vi "Autonomous Independent.vi"() -> ()   [LabVIEW 2014]
doc: "This VI is called when autonomous begins, and will automatically be terminated when autonomous ends. You can carry out timed or sensor driven robot movement independently without needing to return to the caller."
uses:
  <vilib>/Rock Robotics/WPI/Relay/WPI_RelayValue.ctl
  AutonEnum.ctl
  AutonEnumGoAround.ctl
  <vilib>/Rock Robotics/WPI/Joystick/WPI_JoystickGetSetRefNum.vi
  Robot Values.vi
  DriveGlobal.vi
  <vilib>/Rock Robotics/WPI/RobotDrive/WPI_RobotDriveArcadeDrive_Standard(NoSaturation).vi
  Auton1ToteEnum.ctl
panel:
  in  "turn output range 5":cluster{"output high":dbl, "output low":dbl}={"output high"=0.6499999999999999, "output low"=-0.65} {"output low" format="%.2f"; "output high" format="%.2f"}
  in  "PID Turn  gains 5":T1={"proportional gain (Kc)"=0.20000000000000004, "integral time (Ti, min)"=0.0, "derivative time (Td, min)"=0.0} {"derivative time (Td, min)" format="%.3f"; "integral time (Ti, min)" format="%.3f"; "proportional gain (Kc)" format="%.3f"}
  out "Total totes 4":i32
  in  "PID Turn  gains 4":T1={"proportional gain (Kc)"=0.20000000000000004, "integral time (Ti, min)"=0.0, "derivative time (Td, min)"=0.0} {"derivative time (Td, min)" format="%.3f"; "integral time (Ti, min)" format="%.3f"; "proportional gain (Kc)" format="%.3f"}
  in  "turn output range 4":cluster{"output high":dbl, "output low":dbl}={"output high"=0.6500000000000001, "output low"=-0.65} {"output low" format="%.2f"; "output high" format="%.2f"}
  out "Total totes 3":i32
  in  "PID Turn  gains 3":T1={"proportional gain (Kc)"=0.05, "integral time (Ti, min)"=0.01, "derivative time (Td, min)"=0.0} {"derivative time (Td, min)" format="%.3f"; "integral time (Ti, min)" format="%.3f"; "proportional gain (Kc)" format="%.3f"}
  in  "turn output range 3":cluster{"output high":dbl, "output low":dbl}={"output high"=0.4, "output low"=-0.4} {"output low" format="%.2f"; "output high" format="%.2f"}
  out "Total totes 2":i32
  in  "PID Turn  gains 2":T1={"proportional gain (Kc)"=0.05, "integral time (Ti, min)"=0.01, "derivative time (Td, min)"=0.0} {"derivative time (Td, min)" format="%.3f"; "integral time (Ti, min)" format="%.3f"; "proportional gain (Kc)" format="%.3f"}
  in  "turn output range 2":cluster{"output high":dbl, "output low":dbl}={"output high"=0.4, "output low"=-0.4} {"output low" format="%.2f"; "output high" format="%.2f"}
  in  "Average gains 2":T1={"proportional gain (Kc)"=0.05, "integral time (Ti, min)"=0.0, "derivative time (Td, min)"=0.0}
  in  "output range":cluster{"output high":dbl, "output low":dbl}={"output high"=0.6, "output low"=-0.6}
  out "Total totes":i32
  out "Totes grabed":i32
  in  "PID Turn  gains":T1={"proportional gain (Kc)"=0.09999999999999999, "integral time (Ti, min)"=0.01, "derivative time (Td, min)"=0.0} {"derivative time (Td, min)" format="%.3f"; "integral time (Ti, min)" format="%.3f"; "proportional gain (Kc)" format="%.3f"}
  in  "turn output range":cluster{"output high":dbl, "output low":dbl}={"output high"=0.7, "output low"=-0.7} {"output low" format="%.2f"; "output high" format="%.2f"}
  in  "Average gains":T1={"proportional gain (Kc)"=0.01, "integral time (Ti, min)"=0.0, "derivative time (Td, min)"=0.0} {"derivative time (Td, min)" format="%.3f"; "integral time (Ti, min)" format="%.4f"; "proportional gain (Kc)" format="%.3f"}
  in  "name or relative path":string
  in  "P2":dbl[][](array[numeric])
  in  "P1":dbl[][](array[numeric])
  out "Current Movement, for debugging":T2 {"Y Joystick Value" scale=1.0..-1.0; "X Joystick Value" scale=-1.0..1.0}
  in  "Array of robot movements":T3(array[cluster]) {"Y Joystick Value" scale=1.0..-1.0; "X Joystick Value" scale=-1.0..1.0}
  # "Be sure to right-click and choose Data Operations>>Make Current Value default if you want to save the array values with the VI"
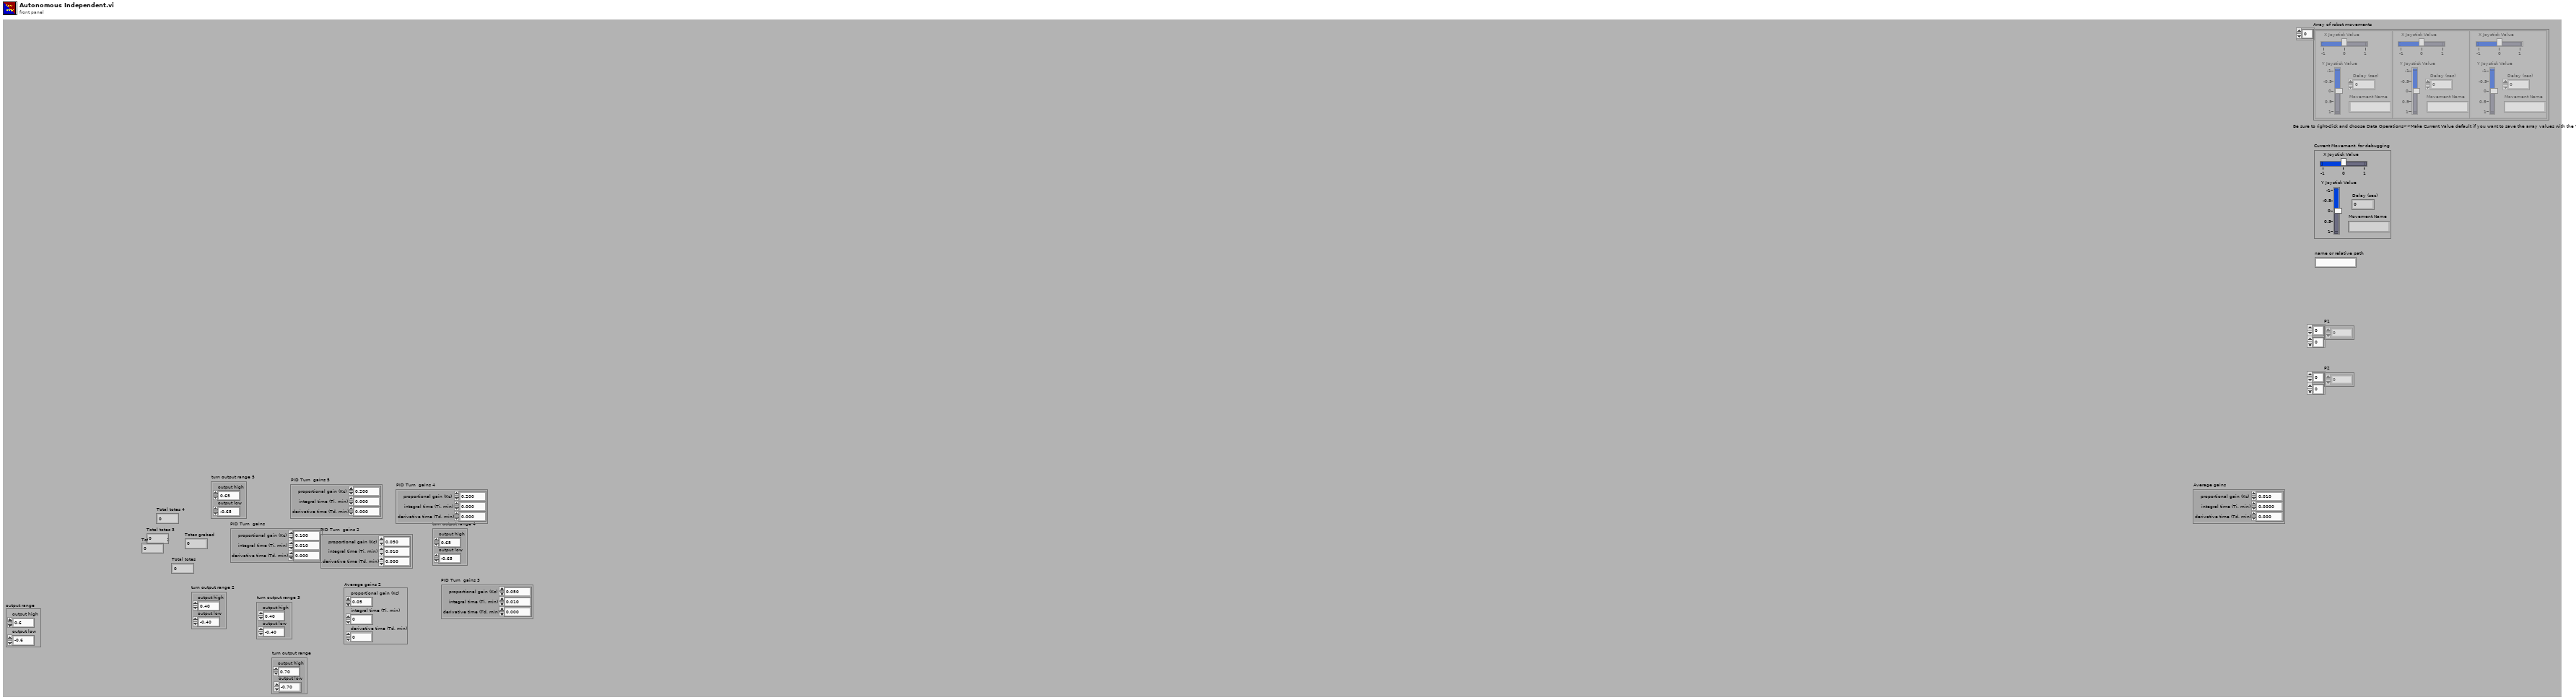
[diagram p1: front panel]
types:
  T1 = cluster{"proportional gain (Kc)":dbl, "integral time (Ti, min)":dbl, "derivative time (Td, min)":dbl}
  T2 = cluster{"X Joystick Value":dbl, "Y Joystick Value":dbl, "Delay (sec)":dbl, "Movement Name":string}
  T3 = cluster{"X Joystick Value":dbl, "Y Joystick Value":dbl, "Delay (sec)":dbl, "Movement Name":string}[]
  T4 = enum16{"Nothing", "Start", "Push", "Finish", "Turn", "Stack"}
  T5 = typedef "WPI_RelayValue.ctl" = enum16{"Off", "On", "Forward", "Reverse"}
  T6 = typedef "AutonEnum.ctl" = enum16{"Go Around", "Nothing", "Start", "Push", "Release Totes", "Turn", "To Auto", "Stack", "Finish"}
  T7 = typedef "AutonEnumGoAround.ctl" = enum16{"Turn Right 1", "Go Straight 1", "Turn Left 1", "Go Straight 2", "Turn Left 2", "Go Straight 3", "Turn Right 3", "Go Straight 4", "Nothing"}
  T8 = typedef "Auton1ToteEnum.ctl" = enum16{"Start", "First Forward", "Get First Tote", "First Pick Up", "Stop"}
  T9 = cluster{"RightMotorSpeed":dbl, "LeftMotorSpeed":dbl}
  T10 = cluster{"Tracking Tote?":bool, "ToteRightSpeed":dbl, "ToteLeftSpeed":dbl, "Drive Encoder reset":bool, "Right Wheel \n(Cm)":dbl, "Left Wheel \n(Cm)":dbl}
  T11 = cluster{"Lift Position":i32, "Lift Speed Override":dbl, "OverrideTele?":bool, "OverrideDash":bool}
  T12 = cluster{"Lift Encoder Height Right (cm)":dbl, "Lift Encoder Height Left (cm)":dbl, "Right Prox":bool, "Left Prox":bool, "Gyro Angle":dbl, "Gyro anglar rate":dbl, "Gyro Reset":bool, "Drive encoder Dash reset":bool}
  T13 = typedef "WPI_JoystickDevRef.ctl" = cluster{"Device":T14}
  T14 = typedef "WPI_JoystickDeviceEnum.ctl" = enum16{"USB 0", "USB 1", "USB 2", "USB 3", "USB 4", "USB 5"}
  T15 = typedef "WPI_RobotDriveDevRef.ctl" = cluster{"DevStatus":errorcluster, "Motors[]":T16[], "Square Inputs":bool, "Max Output":dbl}
  T16 = typedef "WPI_MotorControlDeviceRef.ctl" = cluster{"DeviceStatus":errorcluster, "Type":T17, "PWM":cluster{"Controller":T18, "PWM Channel":T19, "DeadBand":T20}, "CAN":cluster{"Device Number":u8, "Control Mode":T21, "Semaphore":T22, "Max Vout":dbl, "TalonSRX Control Mode":T23}, "Invert":bool, "TransformRef":T24, "InvTransformRef":T24}
  T17 = typedef "WPI_MotorControlType.ctl" = enum16{"PWM", "CAN", "CANTalonSRX"}
  T18 = typedef "FPGA_TypedefDigitalModule.ctl" = enum16{"Controller 1"}
  T19 = typedef "FPGA_DIOPWMChannel.ctl" = enum8{"PWM 0", "PWM 1", "PWM 2", "PWM 3", "PWM 4", "PWM 5", "PWM 6", "PWM 7", "PWM 8", "PWM 9", "PWM MXP 0", "PWM MXP 1", "PWM MXP 2", "PWM MXP 3", "PWM MXP 4", "PWM MXP 5", "PWM MXP 6", "PWM MXP 7", "PWM MXP 8", "PWM MXP 9", "Invalid"}
  T20 = typedef "WPI_PWMDeadband.ctl" = cluster{"Name":string, "maxPositivePwm":i32, "minPositivePwm":i32, "centerPwm":i32, "maxNegativePwm":i32, "minNegativePwm":i32, "angularRange":u16}
  T21 = typedef "WPI_CANJaguar_ControlMode.ctl" = enum8{"Percent VBus", "Current", "Speed", "Position", "Voltage"}
  T22 = typedef "Semaphore RefNum" = refnum<k1>
  T23 = typedef "WPI_CANTalonSRX_APIControlMode.ctl" = enum8{"Percent VBus", "Speed", "Position", "Slave", "Unchanged / Invalid"}
  T24 = typedef "WPI_PWMTransform_ConPane.ctl" = refnum<vi>
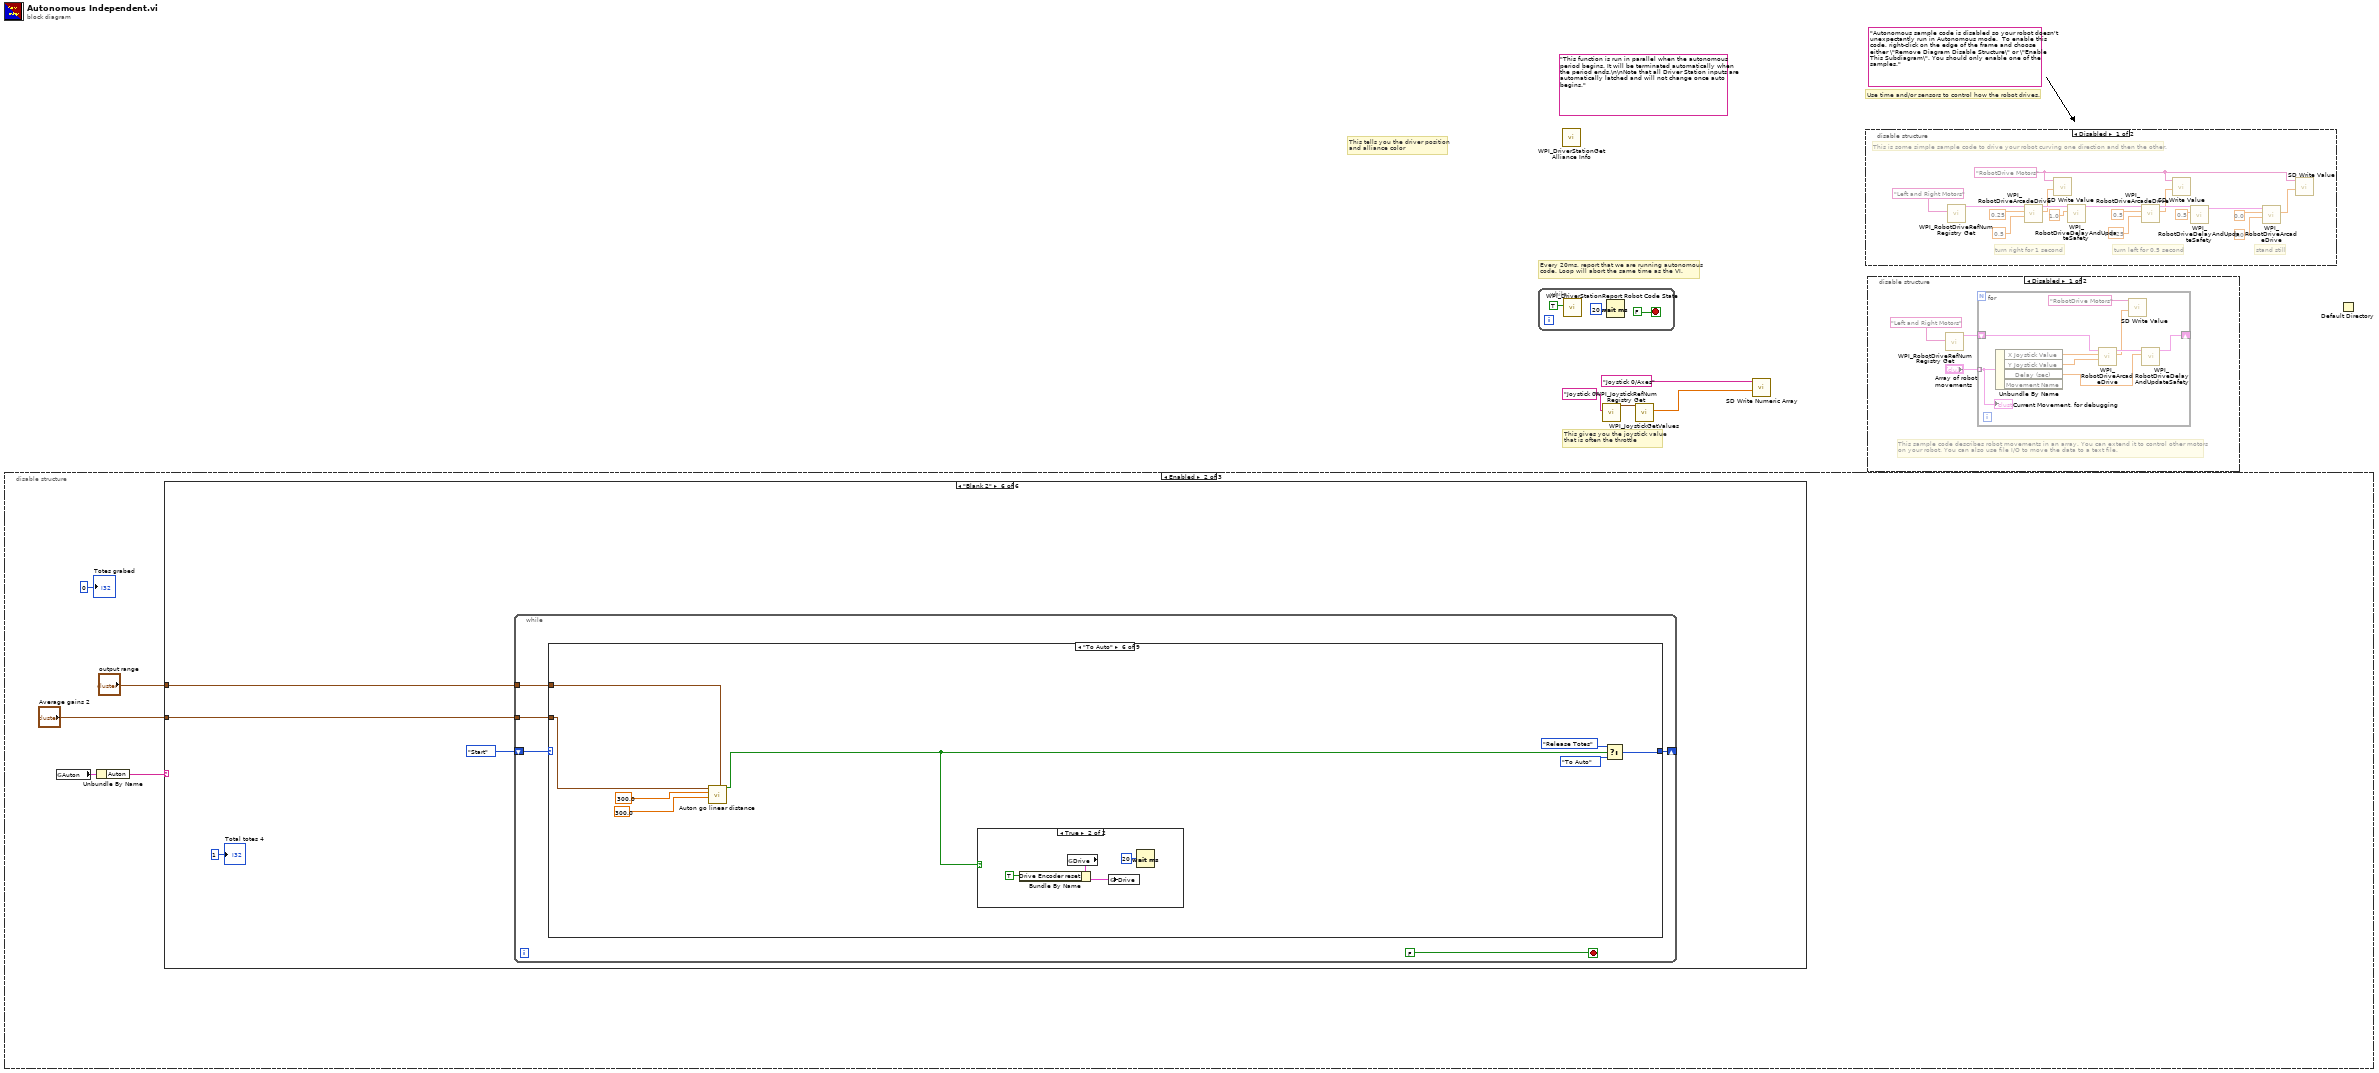
[diagram p0: block diagram]
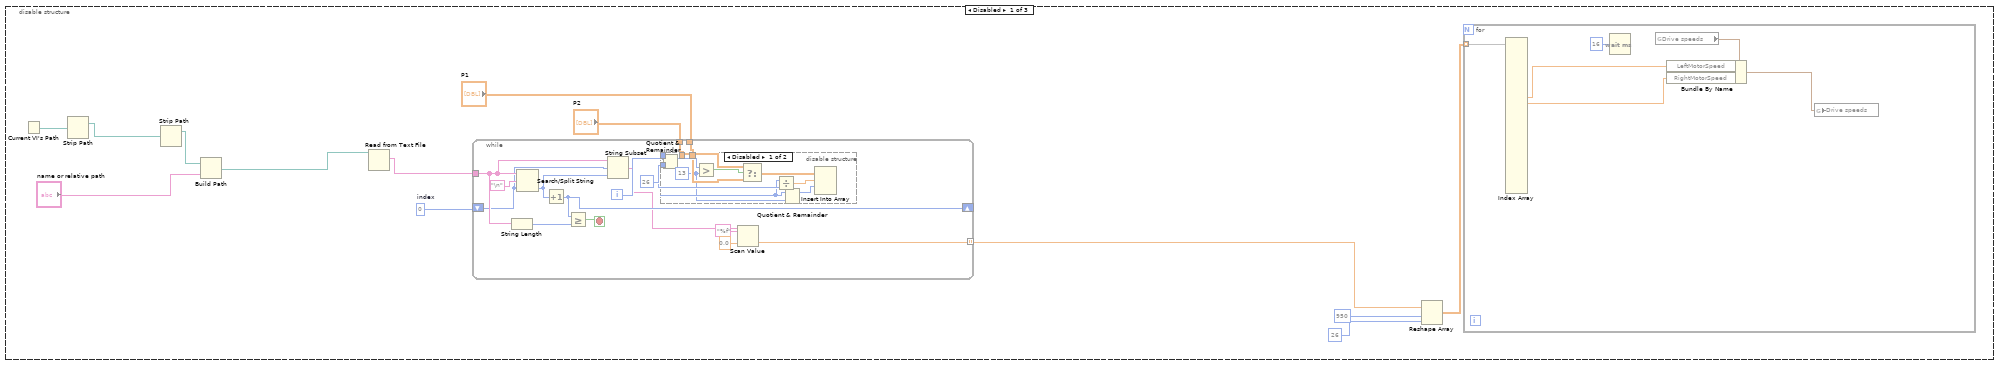
[diagram p2: hidden frame]
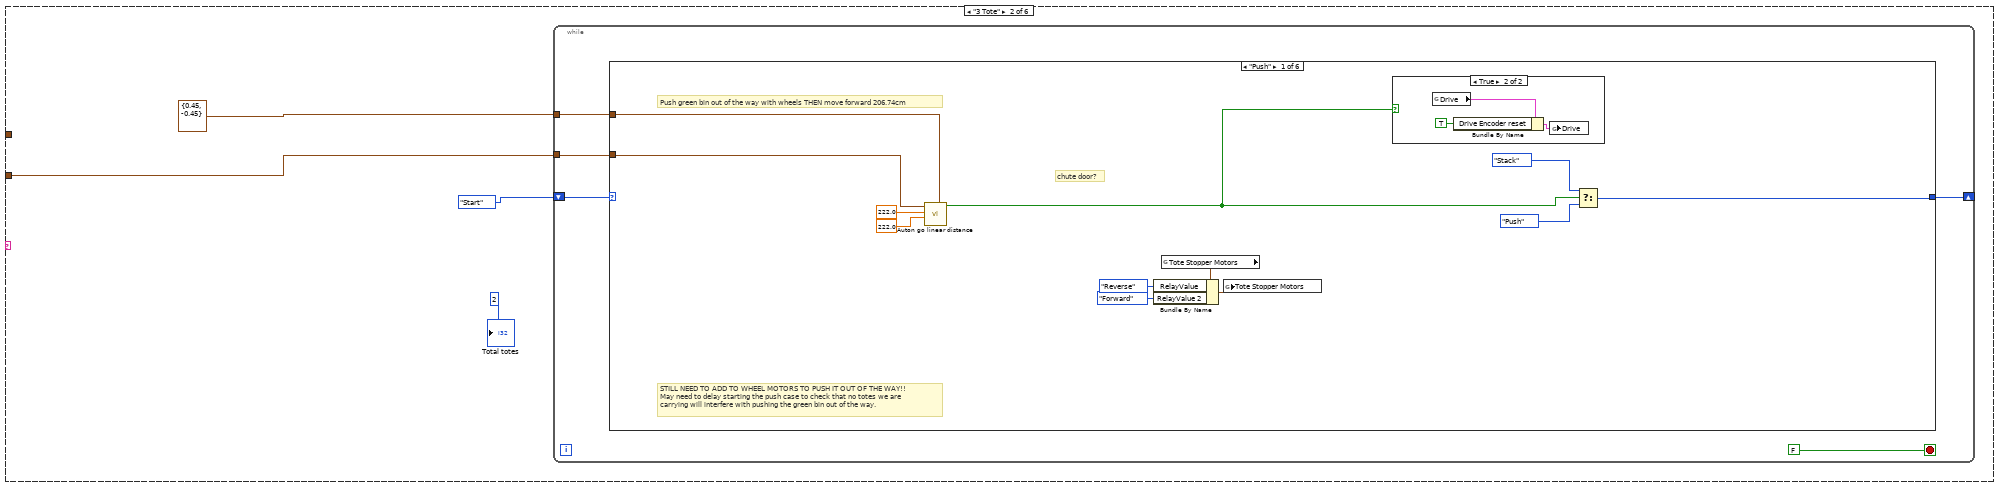
[diagram p5: hidden frame]
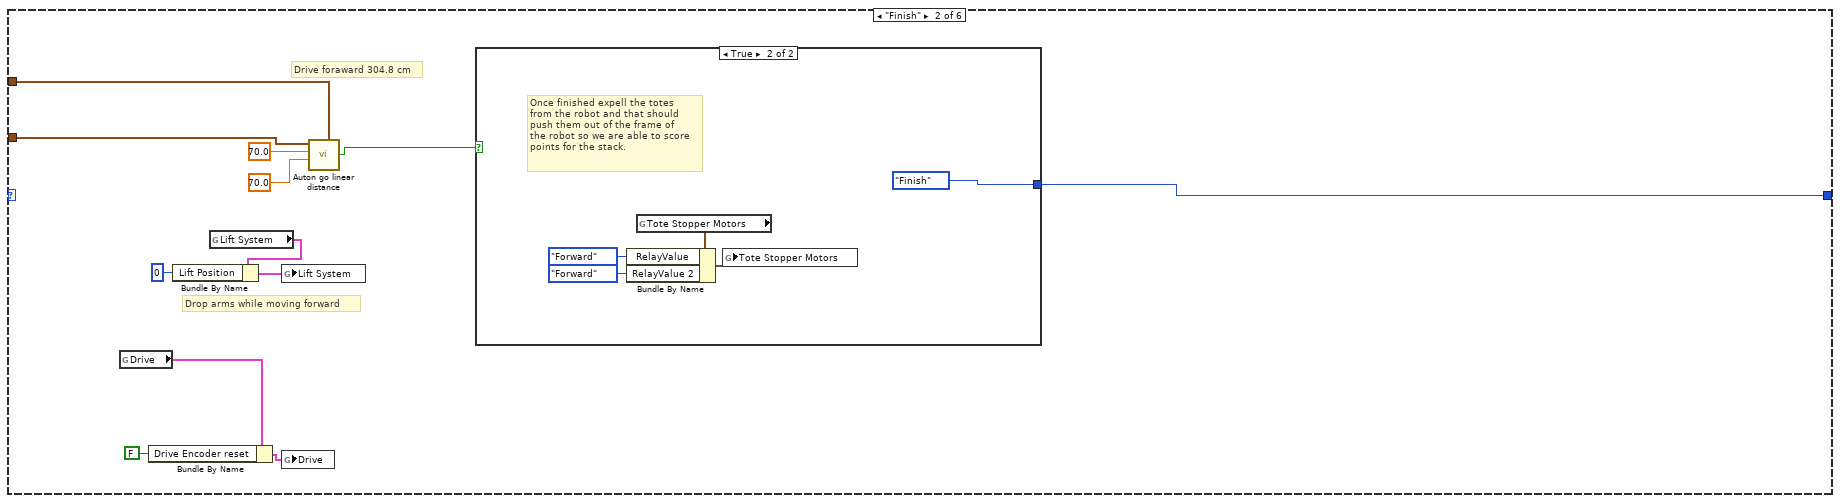
[diagram p7: hidden frame]
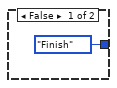
[diagram p8: hidden frame]
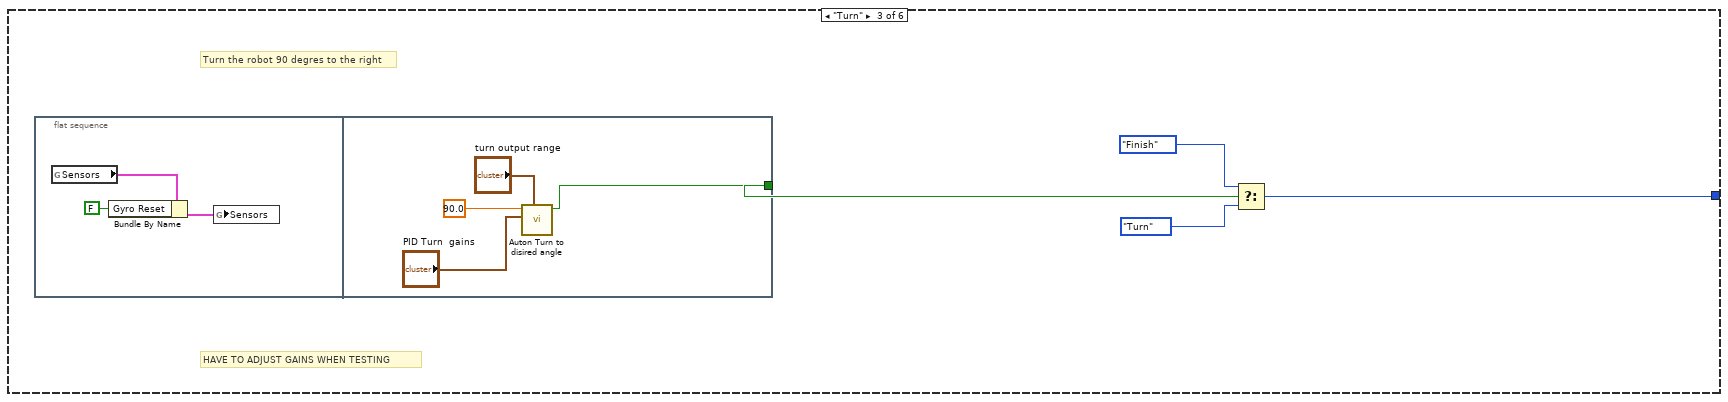
[diagram p9: hidden frame]
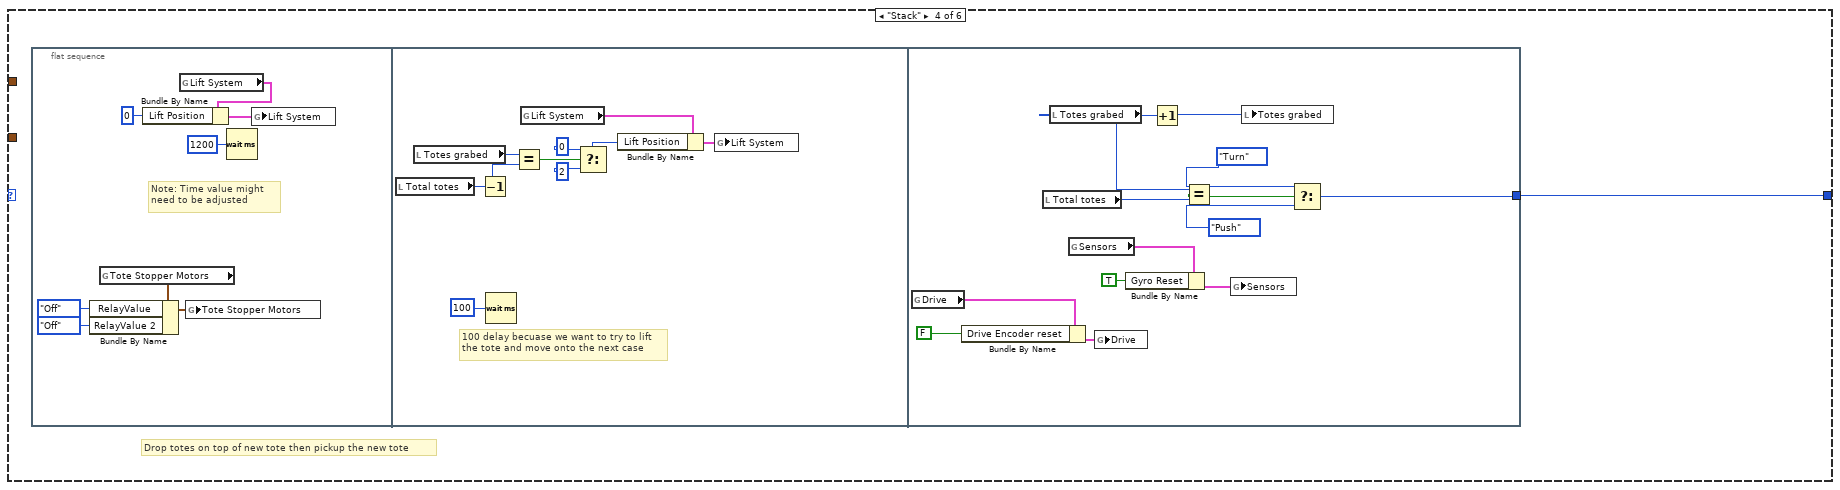
[diagram p10: hidden frame]
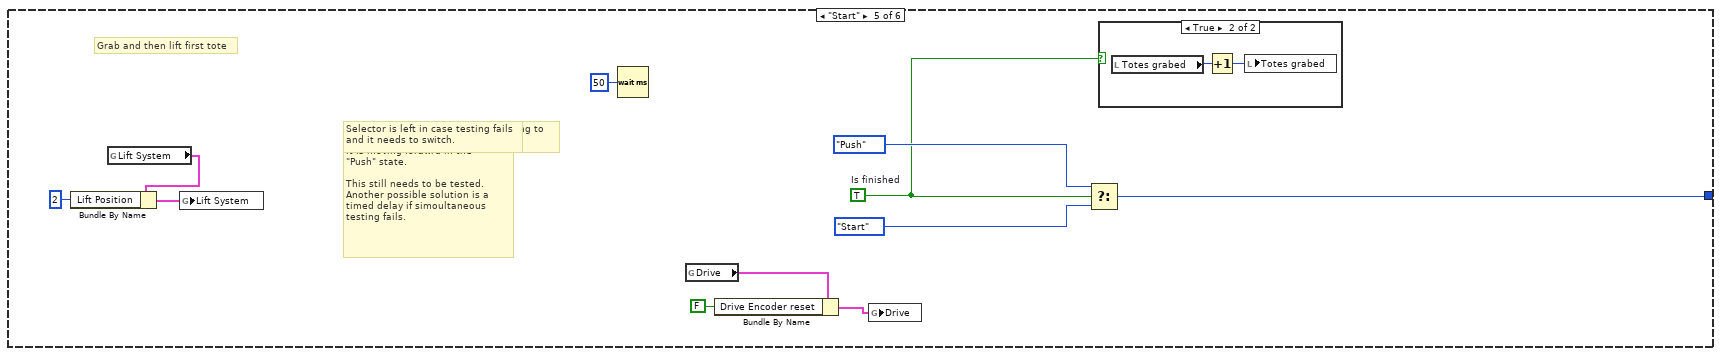
[diagram p11: hidden frame]
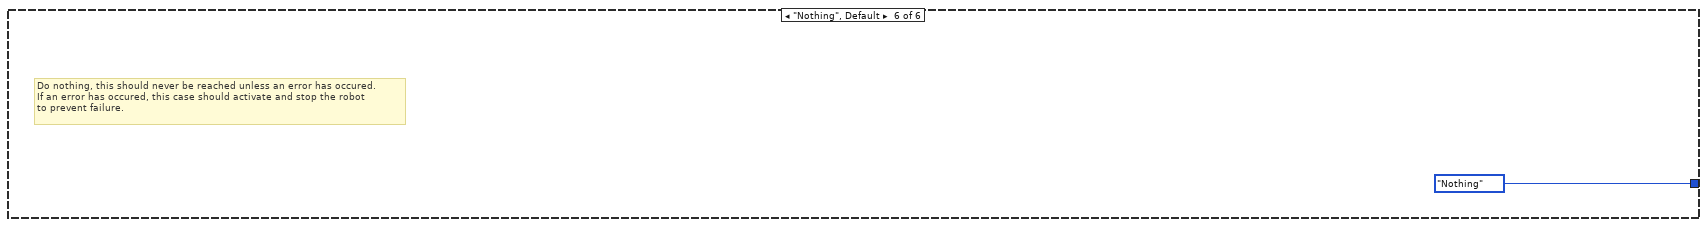
[diagram p13: hidden frame]
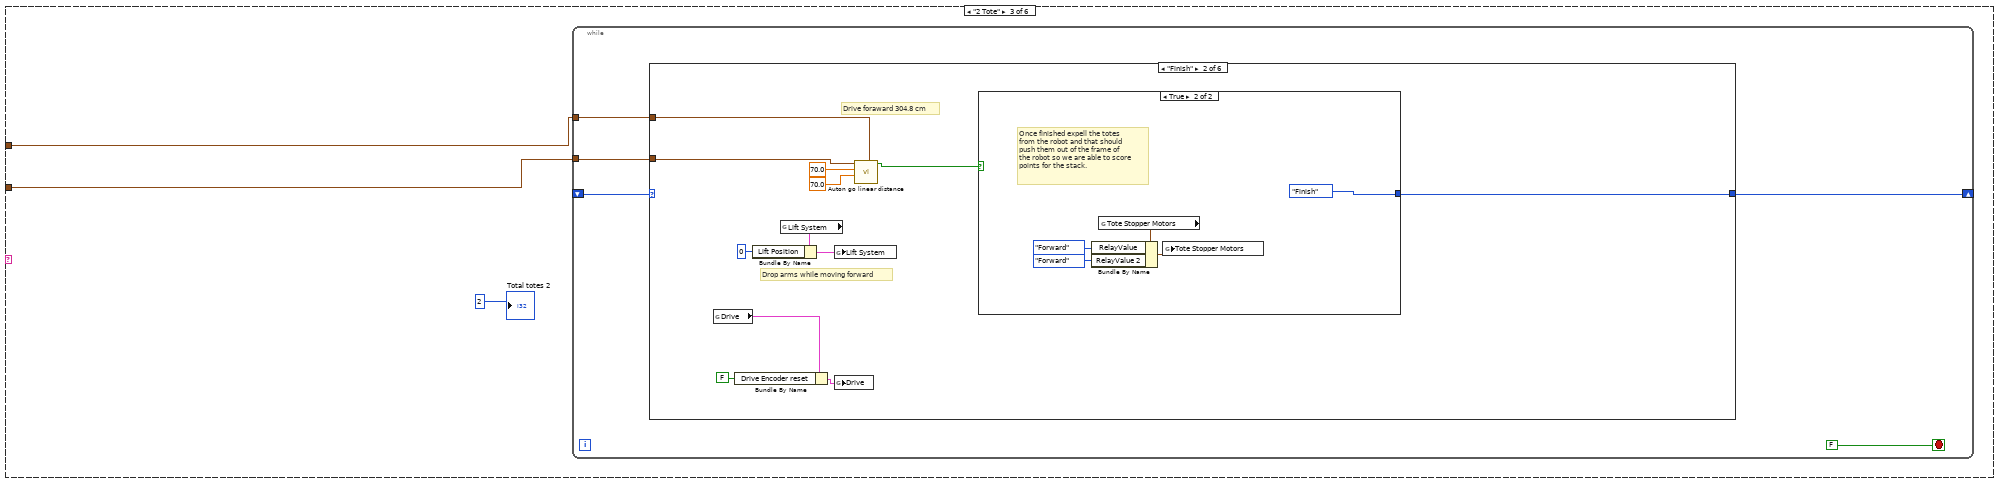
[diagram p14: hidden frame]
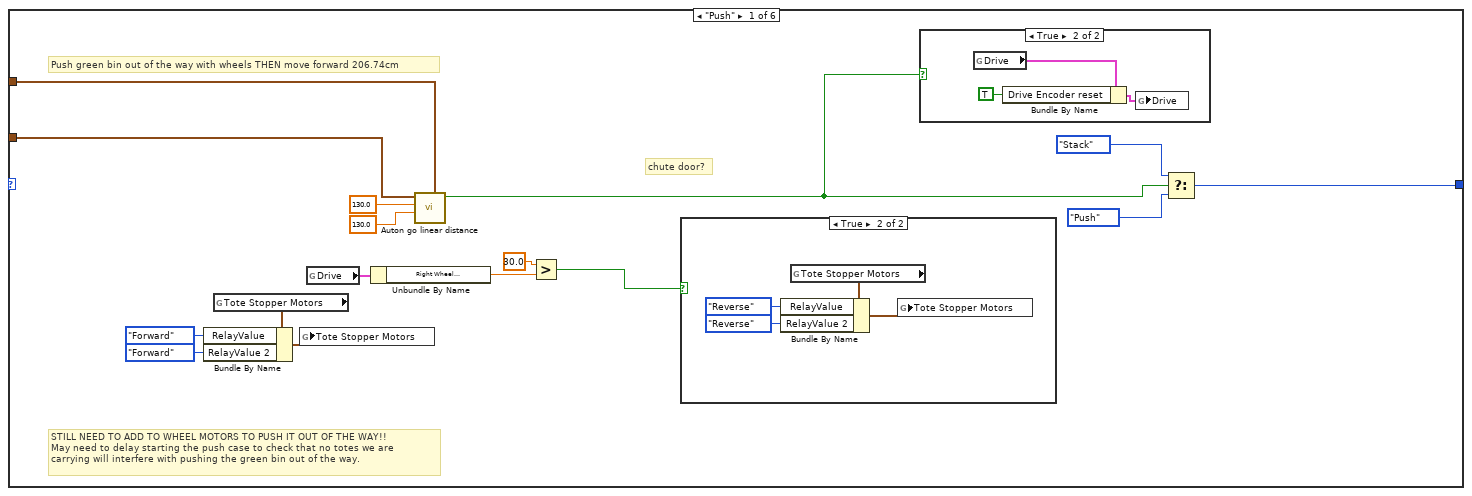
[diagram p15: hidden frame]
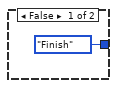
[diagram p18: hidden frame]
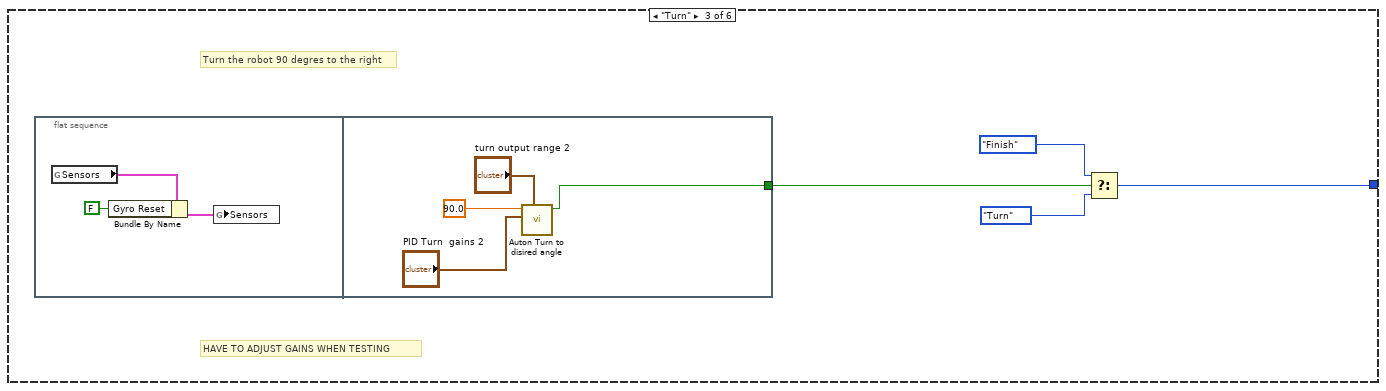
[diagram p19: hidden frame]
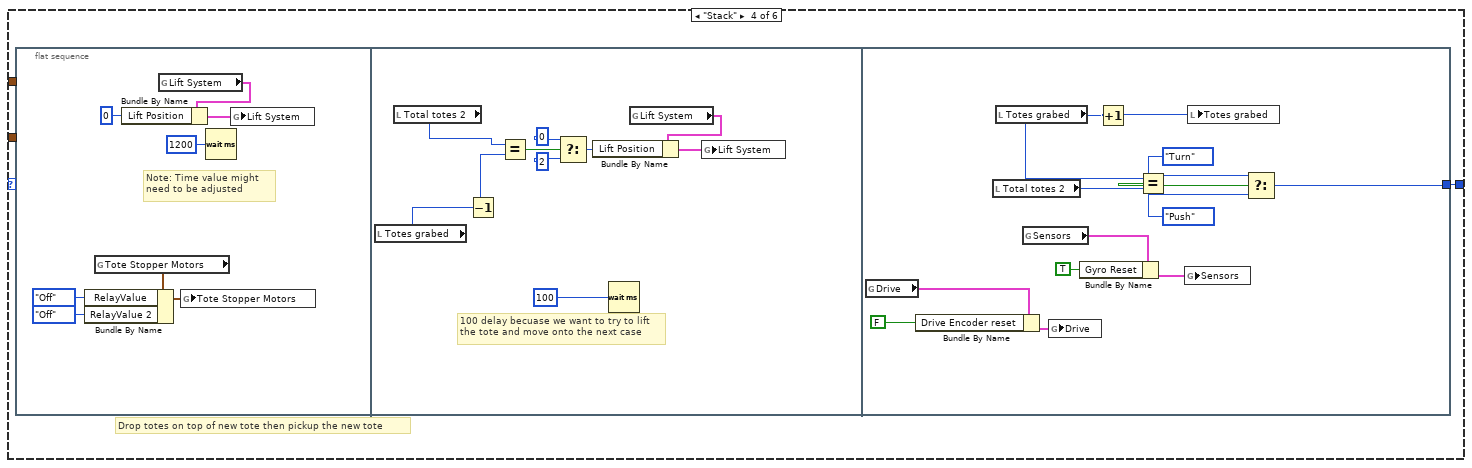
[diagram p20: hidden frame]
diagram:
  (unwired) "Autonomous sample code is disabled so your robot doesn't unexpectantly run in Autonomous mode.  To enable this code, right-click on the edge of the frame and choose either \"Remove Diagram Disable Structure\" or \"Enable This Subdiagram\". You should only enable one of the samples."
  (unwired) "This function is run in parallel when the autonomous period begins. It will be terminated automatically when the period ends.\n\nNote that all Driver Station inputs are automatically latched and will not change once auto begins."
  # "Every 20ms, report that we are running autonomous\ncode. Loop will abort the same time as the VI."
  # "This gives you the joystick value\nthat is often the throttle"
  # "Use time and/or sensors to control how the robot drives."
  # "This tells you the driver position\nand alliance color"
  n1 = disable-structure shown="Enabled" {
    frame Disabled {
      w16 = 0  # index
      n2 = Current VI's Path() -> (path=w10:path)
      n3 = Strip Path(path=w10) -> (stripped path=w9:path)  [unwired: 1 out]
      n4 = Strip Path(path=w9) -> (stripped path=w8:path)  [unwired: 1 out]
      n5 = Build Path(base path=w8, name or relative path="name or relative path") -> (appended path=w7:path)
      n6 = Read from Text File(file (use dialog)=w7) -> (text=w17:string)  [unwired: 3 in, 3 out]
      n7 = while {
        tunnel: w17 -> [w34]
        shift-right: [w35] -> _
        shift-left: w16 -> [w33]
        tunnel: "P1" -> [w30]
        tunnel: "P2" -> [w31]
        tunnel: [w27] -> w13 mode=indexing
        i -> [w28]
        stop <- w37 stop-if-true
        n8 = String Length(string=w34) -> (length=w38:i32)
        n9 = Search/Split String(string=w34, search string/char (-)="\n", offset (0)=w33) -> (offset of match=w32:i32)  [unwired: 2 out]
        n10 = Increment(x=w32) -> (x+1=w35:i32)
        n11 = Greater Or Equal?(x=w35, y=w38) -> (x >= y?=w37:bool)
        n12 = String Subset(string=w34, offset (0)=w33, length (rest)=w32) -> (substring=w26:string)
        n13 = disable-structure shown="Disabled" {
          disable-tunnel: w31 -> [w46 _]
          disable-tunnel: w30 -> [w45 _]
          disable-tunnel: 26 ("y") -> [w42 _]
          disable-tunnel: w28 -> [w40 _]
          frame Disabled {
            w39 = 13 ("y")
            n14 = Quotient & Remainder(x=w40, y=w42) -> (x-y*floor(x/y)=w48:i32)  [unwired: 1 out]
            n15 = Greater?(x=w48, y=w39) -> (0:w47:bool)
            n16 = Select(t=w46, s=w47, f=w45) -> (s? t:f=w44:dbl[][])
            n17 = Divide(x=w40, y=w42) -> (x/y=w43:dbl)
            n18 = Quotient & Remainder(x=w40, y=w39) -> (x-y*floor(x/y)=w41:i32)  [unwired: 1 out]
            n19 = Insert Into Array(array=w44, index (row)=w43, index (col)=w41) -> ()  [unwired: 1 in, 1 out]
          }
          frame Enabled {
          }
        }
        n20 = Scan Value(string=w26, format string="%f", default (0 dbl)=0.0 ("default (0 I32)")) -> (value=w27:dbl)  [unwired: 1 out]
      }
      n21 = Reshape Array(w13, 950 ("dimension size"), 26 ("dimension size")) -> (w5:dbl[][])
      n22 = for {
        tunnel: w5 -> [w23] mode=indexing
        n23 = Index Array(array=w23) -> (element #9=w21:dbl, element #10=w20:dbl)  [unwired: 26 in, 24 out]
        n24 = Wait (ms)(milliseconds to wait=u32 16) -> ()  [unwired: 1 out]
        n25 = global read "DriveGlobal.vi" "Drive speeds"() -> (w19:T9)
        n26 = Bundle By Name(cluster=w19, "LeftMotorSpeed"=w21, "RightMotorSpeed"=w20) -> (w18:T9)
        n27 = global write "DriveGlobal.vi" "Drive speeds"(w18) -> ()
      }
    }
    frame Enabled {
      n28 = global read "Robot Values.vi" "Auton"() -> (w50:cluster{"Auton":string})
      n29 = Unbundle By Name(w50) -> ("Auton"=w49:string)
      n30 = case shown="\"Blank 2\"" w49 {
        tunnel: "Average gains 2" -> [_ w54 w153 w260 w372 w379]
        tunnel: "output range" -> [_ _ w154 w259 w371 w380]
        frame "False", Default {
        }
        frame "3 Tote" {
          n31 = while {
            shift-right: [w61] -> _
            shift-left: T4."Start" -> [w62]
            tunnel: w54 -> [w59]
            tunnel: cluster{"output high":dbl, "output low":dbl} {"output high"=0.45, "output low"=-0.45} ("output range") -> [w58]
            stop <- FALSE stop-if-true
            n32 = case shown="\"Push\"" w62 {
              tunnel: [w72 w81 w97 w107 w147 T4."Nothing"] -> w61
              tunnel: w59 -> [w70 w86 _ _ _ _]
              tunnel: w58 -> [w71 w87 _ _ _ _]
              frame "Push" {
                # "chute door?"
                # "STILL NEED TO ADD TO WHEEL MOTORS TO PUSH IT OUT OF THE WAY!!\nMay need to delay starting the push case to check that no totes we are \ncarrying will interfere with pushing the green bin out of the way."
                # "Push green bin out of the way with wheels THEN move forward 206.74cm"
                n33 = call "Auton go linear distance.vi"("Average gains"=w70, "PID setpoint"=222.0, "Goal"=222.0, "output range"=w71) -> ("Done?"=w68:bool)  [unwired: 4 in]
                n34 = global read "Robot Values.vi" "Tote Stopper Motors"() -> (w64:cluster{"RelayValue":T5, "RelayValue 2":T5})
                n35 = Bundle By Name(cluster=w64, "RelayValue"=WPI_RelayValue."Reverse", "RelayValue 2"=WPI_RelayValue."Forward") -> (w63:cluster{"RelayValue":T5, "RelayValue 2":T5})
                n36 = global write "Robot Values.vi" "Tote Stopper Motors"(w63) -> ()
                n37 = case shown="True" w68 {
                  frame False {
                  }
                  frame True {
                    n38 = global read "Robot Values.vi" "Drive"() -> (w76:T10)
                    n39 = Bundle By Name(cluster=w76, "Drive Encoder reset"=TRUE) -> (w77:T10)
                    n40 = global write "Robot Values.vi" "Drive"(w77) -> ()
                  }
                }
                n41 = Select(t=T4."Stack", s=w68, f=T4."Push") -> (s? t:f=w72:T4)
              }
              frame "Finish" {
                # "Drop arms while moving forward"
                # "Drive foraward 304.8 cm"
                n42 = global read "Robot Values.vi" "Drive"() -> (w83:T10)
                n43 = Bundle By Name(cluster=w83, "Drive Encoder reset"=FALSE) -> (w84:T10)
                n44 = global read "Robot Values.vi" "Lift System"() -> (w79:T11)
                n45 = Bundle By Name(cluster=w79, "Lift Position"=0) -> (w80:T11)
                n46 = global write "Robot Values.vi" "Lift System"(w80) -> ()
                n47 = global write "Robot Values.vi" "Drive"(w84) -> ()
                n48 = call "Auton go linear distance.vi"("Average gains"=w86, "PID setpoint"=70.0, "Goal"=70.0, "output range"=w87) -> ("Done?"=w85:bool)  [unwired: 4 in]
                n49 = case shown="True" w85 {
                  tunnel: [T4."Finish" T4."Finish"] -> w81
                  frame False {
                  }
                  frame True {
                    # "Once finished expell the totes\nfrom the robot and that should\npush them out of the frame of\nthe robot so we are able to score\npoints for the stack."
                    n50 = global read "Robot Values.vi" "Tote Stopper Motors"() -> (w93:cluster{"RelayValue":T5, "RelayValue 2":T5})
                    n51 = Bundle By Name(cluster=w93, "RelayValue"=WPI_RelayValue."Forward", "RelayValue 2"=WPI_RelayValue."Forward") -> (w94:cluster{"RelayValue":T5, "RelayValue 2":T5})
                    n52 = global write "Robot Values.vi" "Tote Stopper Motors"(w94) -> ()
                  }
                }
              }
              frame "Turn" {
                # "HAVE TO ADJUST GAINS WHEN TESTING"
                # "Turn the robot 90 degres to the right"
                n53 = flat-sequence {
                  tunnel: [w103] -> w96
                  frame #0 {
                    n54 = global read "Robot Values.vi" "Sensors"() -> (w101:T12)
                    n55 = Bundle By Name(cluster=w101, "Gyro Reset"=FALSE) -> (w100:T12)
                    n56 = global write "Robot Values.vi" "Sensors"(w100) -> ()
                  }
                  frame #1 {
                    n57 = call "Auton Turn to disired angle.vi"("Power output range"="turn output range", "PID Turn  gains"="PID Turn  gains", "Angle setpoint"=90.0) -> ("In Range?"=w103:bool)  [unwired: 8 in]
                  }
                }
                n58 = Select(t=T4."Finish", s=w96, f=T4."Turn") -> (s? t:f=w97:T4)
              }
              frame "Stack" {
                # "Drop totes on top of new tote then pickup the new tote"
                n59 = flat-sequence {
                  tunnel: [w138] -> w107
                  frame #0 {
                    # "Note: Time value might \nneed to be adjusted"
                    n60 = global read "Robot Values.vi" "Tote Stopper Motors"() -> (w110:cluster{"RelayValue":T5, "RelayValue 2":T5})
                    n61 = Bundle By Name(cluster=w110, "RelayValue"=WPI_RelayValue."Off", "RelayValue 2"=WPI_RelayValue."Off") -> (w111:cluster{"RelayValue":T5, "RelayValue 2":T5})
                    n62 = global read "Robot Values.vi" "Lift System"() -> (w114:T11)
                    n63 = Bundle By Name(cluster=w114, "Lift Position"=0) -> (w113:T11)
                    n64 = global write "Robot Values.vi" "Tote Stopper Motors"(w111) -> ()
                    n65 = Wait (ms)(milliseconds to wait=u32 1200) -> ()  [unwired: 1 out]
                    n66 = global write "Robot Values.vi" "Lift System"(w113) -> ()
                  }
                  frame #1 {
                    # "100 delay becuase we want to try to lift\nthe tote and move onto the next case"
                    n67 = local read "Total totes"() -> (w118:i32)
                    n68 = local read "Totes grabed"() -> (w116:i32)
                    n69 = Decrement(x=w118) -> (x-1=w117:i32)
                    n70 = Wait (ms)(milliseconds to wait=u32 100) -> ()  [unwired: 1 out]
                    n71 = Equal?(x=w116, y=w117) -> (x = y?=w122:bool)
                    n72 = global read "Robot Values.vi" "Lift System"() -> (w124:T11)
                    n73 = Select(t=0 ("Lift Position"), s=w122, f=2 ("Lift Position")) -> (s? t:f=w119:i32)
                    n74 = Bundle By Name(cluster=w124, "Lift Position"=w119) -> (w125:T11)
                    n75 = global write "Robot Values.vi" "Lift System"(w125) -> ()
                  }
                  frame #2 {
                    n76 = global read "Robot Values.vi" "Drive"() -> (w127:T10)
                    n77 = Bundle By Name(cluster=w127, "Drive Encoder reset"=FALSE) -> (w128:T10)
                    n78 = local read "Total totes"() -> (w135:i32)
                    n79 = local read "Totes grabed"() -> (w137:i32)
                    n80 = global read "Robot Values.vi" "Sensors"() -> (w130:T12)
                    n81 = global write "Robot Values.vi" "Drive"(w128) -> ()
                    n82 = Bundle By Name(cluster=w130, "Gyro Reset"=TRUE) -> (w131:T12)
                    n83 = Increment(x=w137) -> (x+1=w136:i32)
                    n84 = Equal?(x=w136, y=w135) -> (x = y?=w133:bool)
                    n85 = global write "Robot Values.vi" "Sensors"(w131) -> ()
                    n86 = local write "Totes grabed"(w136) -> ()
                    n87 = Select(t=T4."Turn", s=w133, f=T4."Push") -> (s? t:f=w138:T4)
                  }
                }
              }
              frame "Start" {
                w146 = TRUE  # Is finished
                # "Selector is left in case testing fails\nand it needs to switch."
                # "Will switch to push state after starting to\nlift the tote."
                # "Is finished is set to true because\nthe robot will lift the tote while\nit is moving forawrd in the\n\"Push\" state.\n\nThis still needs to be tested.\nAnother possible solution is a\ntimed delay if simoultaneous\ntesting fails."
                # "Grab and then lift first tote"
                n88 = global read "Robot Values.vi" "Lift System"() -> (w144:T11)
                n89 = Bundle By Name(cluster=w144, "Lift Position"=2) -> (w145:T11)
                n90 = global write "Robot Values.vi" "Lift System"(w145) -> ()
                n91 = Wait (ms)(milliseconds to wait=u32 50) -> ()  [unwired: 1 out]
                n92 = global read "Robot Values.vi" "Drive"() -> (w141:T10)
                n93 = Bundle By Name(cluster=w141, "Drive Encoder reset"=FALSE) -> (w142:T10)
                n94 = global write "Robot Values.vi" "Drive"(w142) -> ()
                n95 = Select(t=T4."Push", s=w146, f=T4."Start") -> (s? t:f=w147:T4)
                n96 = case shown="True" w146 {
                  frame False {
                  }
                  frame True {
                    n97 = local read "Totes grabed"() -> (w151:i32)
                    n98 = Increment(x=w151) -> (x+1=w150:i32)
                    n99 = local write "Totes grabed"(w150) -> ()
                  }
                }
              }
              frame "Nothing", Default {
                # "Do nothing, this should never be reached unless an error has occured.\nIf an error has occured, this case should activate and stop the robot\nto prevent failure."
              }
            }
          }
          "Total totes" <- 2 ("Total totes")
        }
        frame "2 Tote" {
          n100 = while {
            shift-right: [w159] -> _
            shift-left: _ -> [w160]
            tunnel: w153 -> [w157]
            tunnel: w154 -> [w156]
            stop <- FALSE stop-if-true
            n101 = case shown="\"Finish\"" w160 {
              tunnel: [w174 w187 w203 w213 w253 T4."Nothing"] -> w159
              tunnel: w157 -> [w172 w192 _ _ _ _]
              tunnel: w156 -> [w173 w193 _ _ _ _]
              frame "Push" {
                # "chute door?"
                # "STILL NEED TO ADD TO WHEEL MOTORS TO PUSH IT OUT OF THE WAY!!\nMay need to delay starting the push case to check that no totes we are \ncarrying will interfere with pushing the green bin out of the way."
                # "Push green bin out of the way with wheels THEN move forward 206.74cm"
                n102 = global read "Robot Values.vi" "Tote Stopper Motors"() -> (w169:cluster{"RelayValue":T5, "RelayValue 2":T5})
                n103 = Bundle By Name(cluster=w169, "RelayValue"=WPI_RelayValue."Forward", "RelayValue 2"=WPI_RelayValue."Forward") -> (w170:cluster{"RelayValue":T5, "RelayValue 2":T5})
                n104 = global write "Robot Values.vi" "Tote Stopper Motors"(w170) -> ()
                n105 = global read "Robot Values.vi" "Drive"() -> (w164:T10)
                n106 = Unbundle By Name(w164) -> ("Right Wheel \n(Cm)"=w162:dbl)
                n107 = call "Auton go linear distance.vi"("Average gains"=w172, "PID setpoint"=130.0, "Goal"=130.0, "output range"=w173) -> ("Done?"=w166:bool)  [unwired: 4 in]
                n108 = Greater?(x=30.0, y=w162) -> (0:w161:bool)
                n109 = case shown="True" w161 {
                  frame False {
                  }
                  frame True {
                    n110 = global read "Robot Values.vi" "Tote Stopper Motors"() -> (w178:cluster{"RelayValue":T5, "RelayValue 2":T5})
                    n111 = Bundle By Name(cluster=w178, "RelayValue"=WPI_RelayValue."Reverse", "RelayValue 2"=WPI_RelayValue."Reverse") -> (w177:cluster{"RelayValue":T5, "RelayValue 2":T5})
                    n112 = global write "Robot Values.vi" "Tote Stopper Motors"(w177) -> ()
                  }
                }
                n113 = case shown="True" w166 {
                  frame False {
                  }
                  frame True {
                    n114 = global read "Robot Values.vi" "Drive"() -> (w182:T10)
                    n115 = Bundle By Name(cluster=w182, "Drive Encoder reset"=TRUE) -> (w183:T10)
                    n116 = global write "Robot Values.vi" "Drive"(w183) -> ()
                  }
                }
                n117 = Select(t=T4."Stack", s=w166, f=T4."Push") -> (s? t:f=w174:T4)
              }
              frame "Finish" {
                # "Drop arms while moving forward"
                # "Drive foraward 304.8 cm"
                n118 = global read "Robot Values.vi" "Drive"() -> (w189:T10)
                n119 = Bundle By Name(cluster=w189, "Drive Encoder reset"=FALSE) -> (w190:T10)
                n120 = global read "Robot Values.vi" "Lift System"() -> (w185:T11)
                n121 = Bundle By Name(cluster=w185, "Lift Position"=0) -> (w186:T11)
                n122 = global write "Robot Values.vi" "Lift System"(w186) -> ()
                n123 = global write "Robot Values.vi" "Drive"(w190) -> ()
                n124 = call "Auton go linear distance.vi"("Average gains"=w192, "PID setpoint"=70.0, "Goal"=70.0, "output range"=w193) -> ("Done?"=w191:bool)  [unwired: 4 in]
                n125 = case shown="True" w191 {
                  tunnel: [T4."Finish" T4."Finish"] -> w187
                  frame False {
                  }
                  frame True {
                    # "Once finished expell the totes\nfrom the robot and that should\npush them out of the frame of\nthe robot so we are able to score\npoints for the stack."
                    n126 = global read "Robot Values.vi" "Tote Stopper Motors"() -> (w199:cluster{"RelayValue":T5, "RelayValue 2":T5})
                    n127 = Bundle By Name(cluster=w199, "RelayValue"=WPI_RelayValue."Forward", "RelayValue 2"=WPI_RelayValue."Forward") -> (w200:cluster{"RelayValue":T5, "RelayValue 2":T5})
                    n128 = global write "Robot Values.vi" "Tote Stopper Motors"(w200) -> ()
                  }
                }
              }
              frame "Turn" {
                # "HAVE TO ADJUST GAINS WHEN TESTING"
                # "Turn the robot 90 degres to the right"
                n129 = flat-sequence {
                  tunnel: [w209] -> w202
                  frame #0 {
                    n130 = global read "Robot Values.vi" "Sensors"() -> (w207:T12)
                    n131 = Bundle By Name(cluster=w207, "Gyro Reset"=FALSE) -> (w206:T12)
                    n132 = global write "Robot Values.vi" "Sensors"(w206) -> ()
                  }
                  frame #1 {
                    n133 = call "Auton Turn to disired angle.vi"("Power output range"="turn output range 2", "PID Turn  gains"="PID Turn  gains 2", "Angle setpoint"=90.0) -> ("In Range?"=w209:bool)  [unwired: 8 in]
                  }
                }
                n134 = Select(t=T4."Finish", s=w202, f=T4."Turn") -> (s? t:f=w203:T4)
              }
              frame "Stack" {
                # "Drop totes on top of new tote then pickup the new tote"
                n135 = flat-sequence {
                  tunnel: [w244] -> w213
                  frame #0 {
                    # "Note: Time value might \nneed to be adjusted"
                    n136 = global read "Robot Values.vi" "Tote Stopper Motors"() -> (w216:cluster{"RelayValue":T5, "RelayValue 2":T5})
                    n137 = Bundle By Name(cluster=w216, "RelayValue"=WPI_RelayValue."Off", "RelayValue 2"=WPI_RelayValue."Off") -> (w217:cluster{"RelayValue":T5, "RelayValue 2":T5})
                    n138 = global read "Robot Values.vi" "Lift System"() -> (w220:T11)
                    n139 = Bundle By Name(cluster=w220, "Lift Position"=0) -> (w219:T11)
                    n140 = global write "Robot Values.vi" "Tote Stopper Motors"(w217) -> ()
                    n141 = Wait (ms)(milliseconds to wait=u32 1200) -> ()  [unwired: 1 out]
                    n142 = global write "Robot Values.vi" "Lift System"(w219) -> ()
                  }
                  frame #1 {
                    # "100 delay becuase we want to try to lift\nthe tote and move onto the next case"
                    n143 = local read "Totes grabed"() -> (w223:i32)
                    n144 = local read "Total totes 2"() -> (w224:i32)
                    n145 = Decrement(x=w223) -> (x-1=w222:i32)
                    n146 = Equal?(x=w224, y=w222) -> (x = y?=w228:bool)
                    n147 = Select(t=0 ("Lift Position"), s=w228, f=2 ("Lift Position")) -> (s? t:f=w225:i32)
                    n148 = Wait (ms)(milliseconds to wait=u32 100) -> ()  [unwired: 1 out]
                    n149 = global read "Robot Values.vi" "Lift System"() -> (w230:T11)
                    n150 = Bundle By Name(cluster=w230, "Lift Position"=w225) -> (w231:T11)
                    n151 = global write "Robot Values.vi" "Lift System"(w231) -> ()
                  }
                  frame #2 {
                    n152 = global read "Robot Values.vi" "Drive"() -> (w235:T10)
                    n153 = Bundle By Name(cluster=w235, "Drive Encoder reset"=FALSE) -> (w236:T10)
                    n154 = local read "Total totes 2"() -> (w243:i32)
                    n155 = local read "Totes grabed"() -> (w232:i32)
                    n156 = global read "Robot Values.vi" "Sensors"() -> (w238:T12)
                    n157 = global write "Robot Values.vi" "Drive"(w236) -> ()
                    n158 = Bundle By Name(cluster=w238, "Gyro Reset"=TRUE) -> (w239:T12)
                    n159 = Increment(x=w232) -> (x+1=w233:i32)
                    n160 = Equal?(x=w232, y=w243) -> (x = y?=w241:bool)
                    n161 = global write "Robot Values.vi" "Sensors"(w239) -> ()
                    n162 = local write "Totes grabed"(w233) -> ()
                    n163 = Select(t=T4."Turn", s=w241, f=T4."Push") -> (s? t:f=w244:T4)
                  }
                }
              }
              frame "Start" {
                w252 = TRUE  # Is finished
                # "Selector is left in case testing fails\nand it needs to switch."
                # "Will switch to push state after starting to\nlift the tote."
                # "Is finished is set to true because\nthe robot will lift the tote while\nit is moving forawrd in the\n\"Push\" state.\n\nThis still needs to be tested.\nAnother possible solution is a\ntimed delay if simoultaneous\ntesting fails."
                # "Grab and then lift first tote"
                n164 = global read "Robot Values.vi" "Lift System"() -> (w250:T11)
                n165 = Bundle By Name(cluster=w250, "Lift Position"=2) -> (w251:T11)
                n166 = global write "Robot Values.vi" "Lift System"(w251) -> ()
                n167 = Wait (ms)(milliseconds to wait=u32 50) -> ()  [unwired: 1 out]
                n168 = global read "Robot Values.vi" "Drive"() -> (w247:T10)
                n169 = Bundle By Name(cluster=w247, "Drive Encoder reset"=FALSE) -> (w248:T10)
                n170 = global write "Robot Values.vi" "Drive"(w248) -> ()
                n171 = Select(t=T4."Push", s=w252, f=T4."Start") -> (s? t:f=w253:T4)
                n172 = case shown="True" w252 {
                  frame False {
                  }
                  frame True {
                    n173 = local read "Totes grabed"() -> (w257:i32)
                    n174 = Increment(x=w257) -> (x+1=w256:i32)
                    n175 = local write "Totes grabed"(w256) -> ()
                  }
                }
              }
              frame "Nothing", Default {
                # "Do nothing, this should never be reached unless an error has occured.\nIf an error has occured, this case should activate and stop the robot\nto prevent failure."
              }
            }
          }
          "Total totes 2" <- 2 ("Total totes")
        }
        frame "1 Tote" {
          n176 = while {
            shift-right: [w266] -> _
            shift-left: T4."Start" -> [w267]
            tunnel: w260 -> [w264]
            tunnel: w259 -> [w263]
            stop <- FALSE stop-if-true
            n177 = case shown="\"Finish\"" w267 {
              tunnel: [w279 w294 w308 w318 w362 T4."Nothing"] -> w266
              tunnel: w264 -> [_ w290 _ _ _ _]
              tunnel: w263 -> [_ _ _ _ _ _]
              frame "Push" {
                # "chute door?"
                # "STILL NEED TO ADD TO WHEEL MOTORS TO PUSH IT OUT OF THE WAY!!\nMay need to delay starting the push case to check that no totes we are \ncarrying will interfere with pushing the green bin out of the way."
                # "Push green bin out of the way with wheels THEN move forward 206.74cm"
                n178 = global read "Robot Values.vi" "Tote Stopper Motors"() -> (w276:cluster{"RelayValue":T5, "RelayValue 2":T5})
                n179 = Bundle By Name(cluster=w276, "RelayValue"=WPI_RelayValue."Forward", "RelayValue 2"=WPI_RelayValue."Forward") -> (w277:cluster{"RelayValue":T5, "RelayValue 2":T5})
                n180 = global write "Robot Values.vi" "Tote Stopper Motors"(w277) -> ()
                n181 = global read "Robot Values.vi" "Drive"() -> (w271:T10)
                n182 = Unbundle By Name(w271) -> ("Right Wheel \n(Cm)"=w269:dbl)
                n183 = call "Auton go linear distance.vi"("PID setpoint"=130.0, "Goal"=130.0) -> ("Done?"=w273:bool)  [unwired: 6 in]
                n184 = Greater?(x=30.0, y=w269) -> (0:w268:bool)
                n185 = case shown="True" w268 {
                  frame False {
                  }
                  frame True {
                    n186 = global read "Robot Values.vi" "Tote Stopper Motors"() -> (w283:cluster{"RelayValue":T5, "RelayValue 2":T5})
                    n187 = Bundle By Name(cluster=w283, "RelayValue"=WPI_RelayValue."Reverse", "RelayValue 2"=WPI_RelayValue."Reverse") -> (w282:cluster{"RelayValue":T5, "RelayValue 2":T5})
                    n188 = global write "Robot Values.vi" "Tote Stopper Motors"(w282) -> ()
                  }
                }
                n189 = case shown="True" w273 {
                  frame False {
                  }
                  frame True {
                    n190 = global read "Robot Values.vi" "Drive"() -> (w287:T10)
                    n191 = Bundle By Name(cluster=w287, "Drive Encoder reset"=TRUE) -> (w288:T10)
                    n192 = global write "Robot Values.vi" "Drive"(w288) -> ()
                  }
                }
                n193 = Select(t=T4."Stack", s=w273, f=T4."Push") -> (s? t:f=w279:T4)
              }
              frame "Finish" {
                # "Russ did this"
                # "Drop arms while moving forward"
                # "Drive foraward 304.8 cm"
                n194 = global read "Robot Values.vi" "Drive"() -> (w296:T10)
                n195 = Bundle By Name(cluster=w296, "Drive Encoder reset"=FALSE) -> (w297:T10)
                n196 = global read "Robot Values.vi" "Lift System"() -> (w292:T11)
                n197 = Bundle By Name(cluster=w292, "Lift Position"=0) -> (w293:T11)
                n198 = global write "Robot Values.vi" "Lift System"(w293) -> ()
                n199 = global write "Robot Values.vi" "Drive"(w297) -> ()
                n200 = call "Auton go linear distance.vi"("Average gains"=w290, "PID setpoint"=452.0, "Goal"=450.0, "output range"=cluster{"output high":dbl, "output low":dbl} {"output high"=0.65, "output low"=-0.65}) -> ("Done?"=w298:bool)  [unwired: 4 in]
                n201 = case shown="True" w298 {
                  tunnel: [T4."Finish" T4."Nothing"] -> w294
                  frame False {
                  }
                  frame True {
                    # "Once finished expell the totes\nfrom the robot and that should\npush them out of the frame of\nthe robot so we are able to score\npoints for the stack."
                    n202 = global read "Robot Values.vi" "Tote Stopper Motors"() -> (w304:cluster{"RelayValue":T5, "RelayValue 2":T5})
                    n203 = Bundle By Name(cluster=w304, "RelayValue"=WPI_RelayValue."Forward", "RelayValue 2"=WPI_RelayValue."Forward") -> (w305:cluster{"RelayValue":T5, "RelayValue 2":T5})
                    n204 = global write "Robot Values.vi" "Tote Stopper Motors"(w305) -> ()
                  }
                }
              }
              frame "Turn" {
                # "HAVE TO ADJUST GAINS WHEN TESTING"
                # "Turn the robot 90 degres to the right"
                n205 = flat-sequence {
                  tunnel: [w314] -> w307
                  frame #0 {
                    n206 = global read "Robot Values.vi" "Sensors"() -> (w312:T12)
                    n207 = Bundle By Name(cluster=w312, "Gyro Reset"=FALSE) -> (w311:T12)
                    n208 = global write "Robot Values.vi" "Sensors"(w311) -> ()
                  }
                  frame #1 {
                    n209 = call "Auton Turn to disired angle.vi"("Power output range"="turn output range 3", "PID Turn  gains"="PID Turn  gains 3", "Angle setpoint"=90.0) -> ("In Range?"=w314:bool)  [unwired: 8 in]
                  }
                }
                n210 = Select(t=T4."Finish", s=w307, f=T4."Turn") -> (s? t:f=w308:T4)
              }
              frame "Stack" {
                # "Drop totes on top of new tote then pickup the new tote"
                n211 = flat-sequence {
                  tunnel: [w349] -> w318
                  frame #0 {
                    # "Note: Time value might \nneed to be adjusted"
                    n212 = global read "Robot Values.vi" "Tote Stopper Motors"() -> (w321:cluster{"RelayValue":T5, "RelayValue 2":T5})
                    n213 = Bundle By Name(cluster=w321, "RelayValue"=WPI_RelayValue."Off", "RelayValue 2"=WPI_RelayValue."Off") -> (w322:cluster{"RelayValue":T5, "RelayValue 2":T5})
                    n214 = global read "Robot Values.vi" "Lift System"() -> (w325:T11)
                    n215 = Bundle By Name(cluster=w325, "Lift Position"=0) -> (w324:T11)
                    n216 = global write "Robot Values.vi" "Tote Stopper Motors"(w322) -> ()
                    n217 = Wait (ms)(milliseconds to wait=u32 1200) -> ()  [unwired: 1 out]
                    n218 = global write "Robot Values.vi" "Lift System"(w324) -> ()
                  }
                  frame #1 {
                    # "100 delay becuase we want to try to lift\nthe tote and move onto the next case"
                    n219 = local read "Total totes 3"() -> (w329:i32)
                    n220 = local read "Totes grabed"() -> (w328:i32)
                    n221 = Decrement(x=w328) -> (x-1=w327:i32)
                    n222 = Equal?(x=w329, y=w327) -> (x = y?=w333:bool)
                    n223 = Select(t=0 ("Lift Position"), s=w333, f=2 ("Lift Position")) -> (s? t:f=w330:i32)
                    n224 = Wait (ms)(milliseconds to wait=u32 100) -> ()  [unwired: 1 out]
                    n225 = global read "Robot Values.vi" "Lift System"() -> (w335:T11)
                    n226 = Bundle By Name(cluster=w335, "Lift Position"=w330) -> (w336:T11)
                    n227 = global write "Robot Values.vi" "Lift System"(w336) -> ()
                  }
                  frame #2 {
                    n228 = global read "Robot Values.vi" "Drive"() -> (w340:T10)
                    n229 = Bundle By Name(cluster=w340, "Drive Encoder reset"=FALSE) -> (w341:T10)
                    n230 = local read "Totes grabed"() -> (w337:i32)
                    n231 = local read "Total totes 3"() -> (w348:i32)
                    n232 = global read "Robot Values.vi" "Sensors"() -> (w343:T12)
                    n233 = global write "Robot Values.vi" "Drive"(w341) -> ()
                    n234 = Bundle By Name(cluster=w343, "Gyro Reset"=TRUE) -> (w344:T12)
                    n235 = Increment(x=w337) -> (x+1=w338:i32)
                    n236 = Equal?(x=w337, y=w348) -> (x = y?=w346:bool)
                    n237 = global write "Robot Values.vi" "Sensors"(w344) -> ()
                    n238 = local write "Totes grabed"(w338) -> ()
                    n239 = Select(t=T4."Turn", s=w346, f=T4."Push") -> (s? t:f=w349:T4)
                  }
                }
              }
              frame "Start" {
                w361 = TRUE  # Is finished
                # "Selector is left in case testing fails\nand it needs to switch."
                # "Will switch to push state after starting to\nlift the tote."
                # "Is finished is set to true because\nthe robot will lift the tote while\nit is moving forawrd in the\n\"Push\" state.\n\nThis still needs to be tested.\nAnother possible solution is a\ntimed delay if simoultaneous\ntesting fails."
                # "Grab and then lift first tote"
                n240 = global read "Robot Values.vi" "Lift System"() -> (w359:T11)
                n241 = Bundle By Name(cluster=w359, "Lift Position"=0) -> (w360:T11)
                n242 = global write "Robot Values.vi" "Lift System"(w360) -> ()
                n243 = global read "Robot Values.vi" "Tote Stopper Motors"() -> (w352:cluster{"RelayValue":T5, "RelayValue 2":T5})
                n244 = Bundle By Name(cluster=w352, "RelayValue"=WPI_RelayValue."Off", "RelayValue 2"=WPI_RelayValue."Off") -> (w353:cluster{"RelayValue":T5, "RelayValue 2":T5})
                n245 = global write "Robot Values.vi" "Tote Stopper Motors"(w353) -> ()
                n246 = Wait (ms)(milliseconds to wait=u32 50) -> ()  [unwired: 1 out]
                n247 = global read "Robot Values.vi" "Drive"() -> (w356:T10)
                n248 = Bundle By Name(cluster=w356, "Drive Encoder reset"=FALSE) -> (w357:T10)
                n249 = global write "Robot Values.vi" "Drive"(w357) -> ()
                n250 = Select(t=T4."Turn", s=w361, f=T4."Start") -> (s? t:f=w362:T4)
                n251 = case shown="True" w361 {
                  frame False {
                  }
                  frame True {
                    n252 = local read "Totes grabed"() -> (w366:i32)
                    n253 = Increment(x=w366) -> (x+1=w365:i32)
                    n254 = local write "Totes grabed"(w365) -> ()
                  }
                }
              }
              frame "Nothing", Default {
                w367 = 0.0
                # "Do nothing, this should never be reached unless an error has occured.\nIf an error has occured, this case should activate and stop the robot\nto prevent failure."
                n255 = global read "DriveGlobal.vi" "Drive speeds"() -> (w368:T9)
                n256 = Bundle By Name(cluster=w368, "RightMotorSpeed"=w367, "LeftMotorSpeed"=w367) -> (w369:T9)
                n257 = global write "DriveGlobal.vi" "Drive speeds"(w369) -> ()
              }
            }
          }
          "Total totes 3" <- 0 ("Total totes")
        }
        frame "Blank 1" {
          n258 = while {
            tunnel: w372 -> [w377]
            tunnel: w371 -> [w376]
            stop <- w373 stop-if-true
            n259 = call "Auton go linear distance.vi"("Average gains"=w377, "PID setpoint"=300.0, "Goal"=300.0, "output range"=w376) -> ("Done?"=w373:bool)  [unwired: 4 in]
          }
        }
        frame "Blank 2" {
          n260 = while {
            shift-right: [w385] -> _
            shift-left: AutonEnum."Start" -> [w386]
            tunnel: w379 -> [w383]
            tunnel: w380 -> [w382]
            stop <- FALSE stop-if-true
            n261 = case shown="\"To Auto\"" w386 {
              tunnel: [w402 w413 w431 w445 w570 w596 AutonEnum."Nothing" w631 AutonEnum."Nothing"] -> w385
              tunnel: w383 -> [w400 w418 _ w450 _ w600 _ _ _]
              tunnel: w382 -> [w401 w419 _ w451 _ w599 _ _ _]
              frame "Push" {
                # "chute door?"
                # "STILL NEED TO ADD TO WHEEL MOTORS TO PUSH IT OUT OF THE WAY!!\nMay need to delay starting the push case to check that no totes we are \ncarrying will interfere with pushing the green bin out of the way."
                # "Push green bin out of the way with wheels THEN move forward 206.74cm"
                n262 = global read "Robot Values.vi" "Tote Stopper Motors"() -> (w397:cluster{"RelayValue":T5, "RelayValue 2":T5})
                n263 = Bundle By Name(cluster=w397, "RelayValue"=WPI_RelayValue."Forward", "RelayValue 2"=WPI_RelayValue."Forward") -> (w398:cluster{"RelayValue":T5, "RelayValue 2":T5})
                n264 = global write "Robot Values.vi" "Tote Stopper Motors"(w398) -> ()
                n265 = global read "Robot Values.vi" "Drive"() -> (w392:T10)
                n266 = Unbundle By Name(w392) -> ("Right Wheel \n(Cm)"=w390:dbl)
                n267 = call "Auton go linear distance.vi"("Average gains"=w400, "PID setpoint"=130.0, "Goal"=130.0, "output range"=w401) -> ("Done?"=w394:bool)  [unwired: 4 in]
                n268 = Greater?(x=30.0, y=w390) -> (0:w389:bool)
                n269 = case shown="True" w389 {
                  frame False {
                  }
                  frame True {
                    n270 = global read "Robot Values.vi" "Tote Stopper Motors"() -> (w404:cluster{"RelayValue":T5, "RelayValue 2":T5})
                    n271 = Bundle By Name(cluster=w404, "RelayValue"=WPI_RelayValue."Reverse", "RelayValue 2"=WPI_RelayValue."Reverse") -> (w403:cluster{"RelayValue":T5, "RelayValue 2":T5})
                    n272 = global write "Robot Values.vi" "Tote Stopper Motors"(w403) -> ()
                  }
                }
                n273 = case shown="True" w394 {
                  frame False {
                  }
                  frame True {
                    n274 = global read "Robot Values.vi" "Drive"() -> (w408:T10)
                    n275 = Bundle By Name(cluster=w408, "Drive Encoder reset"=TRUE) -> (w409:T10)
                    n276 = global write "Robot Values.vi" "Drive"(w409) -> ()
                  }
                }
                n277 = Select(t=AutonEnum."Stack", s=w394, f=AutonEnum."Push") -> (s? t:f=w402:T6)
              }
              frame "Finish" {
                # "Drop arms while moving forward"
                # "Drive foraward 304.8 cm"
                n278 = global read "Robot Values.vi" "Drive"() -> (w415:T10)
                n279 = Bundle By Name(cluster=w415, "Drive Encoder reset"=FALSE) -> (w416:T10)
                n280 = global read "Robot Values.vi" "Lift System"() -> (w411:T11)
                n281 = Bundle By Name(cluster=w411, "Lift Position"=0) -> (w412:T11)
                n282 = global write "Robot Values.vi" "Lift System"(w412) -> ()
                n283 = global write "Robot Values.vi" "Drive"(w416) -> ()
                n284 = call "Auton go linear distance.vi"("Average gains"=w418, "PID setpoint"=70.0, "Goal"=70.0, "output range"=w419) -> ("Done?"=w417:bool)  [unwired: 4 in]
                n285 = case shown="True" w417 {
                  tunnel: [AutonEnum."Finish" AutonEnum."Finish"] -> w413
                  frame False {
                  }
                  frame True {
                    # "Once finished expell the totes\nfrom the robot and that should\npush them out of the frame of\nthe robot so we are able to score\npoints for the stack."
                    n286 = global read "Robot Values.vi" "Tote Stopper Motors"() -> (w426:cluster{"RelayValue":T5, "RelayValue 2":T5})
                    n287 = Bundle By Name(cluster=w426, "RelayValue"=WPI_RelayValue."Forward", "RelayValue 2"=WPI_RelayValue."Forward") -> (w427:cluster{"RelayValue":T5, "RelayValue 2":T5})
                    n288 = global write "Robot Values.vi" "Tote Stopper Motors"(w427) -> ()
                  }
                }
              }
              frame "Turn" {
                # "HAVE TO ADJUST GAINS WHEN TESTING"
                # "Turn the robot 90 degres to the right"
                n289 = flat-sequence {
                  tunnel: [w435] -> w430
                  frame #0 {
                    n290 = global read "Robot Values.vi" "Sensors"() -> (w433:T12)
                    n291 = Bundle By Name(cluster=w433, "Gyro Reset"=FALSE) -> (w432:T12)
                    n292 = global write "Robot Values.vi" "Sensors"(w432) -> ()
                  }
                  frame #1 {
                    n293 = call "Auton Turn to disired angle.vi"("Power output range"="turn output range 4", "PID Turn  gains"="PID Turn  gains 4", "Angle setpoint"=45.0) -> ("In Range?"=w435:bool)  [unwired: 8 in]
                    n294 = case shown="True" w435 {
                      frame False {
                      }
                      frame True {
                        n295 = Wait (ms)(milliseconds to wait=u32 20) -> ()  [unwired: 1 out]
                        n296 = global read "Robot Values.vi" "Drive"() -> (w441:T10)
                        n297 = Bundle By Name(cluster=w441, "Drive Encoder reset"=TRUE) -> (w442:T10)
                        n298 = global write "Robot Values.vi" "Drive"(w442) -> ()
                      }
                    }
                  }
                }
                n299 = Select(t=AutonEnum."To Auto", s=w430, f=AutonEnum."Turn") -> (s? t:f=w431:T6)
              }
              frame "Go Around" {
                n300 = while {
                  shift-right: [w457] -> _
                  shift-left: AutonEnumGoAround."Turn Right 1" -> [w458]
                  tunnel: w451 -> [w456]
                  tunnel: w450 -> [w455]
                  tunnel: [w454] -> w448
                  tunnel: "turn output range 5" -> [w453]
                  tunnel: "PID Turn  gains 5" -> [w452]
                  stop <- w454 stop-if-true
                  n301 = case shown="\"Turn Left 2\"" w458 {
                    tunnel: [w464 w478 w489 w500 w514 w535 w546 w562 AutonEnumGoAround."Nothing"] -> w457
                    tunnel: w456 -> [_ w480 _ w501 _ _ _ w563 _]
                    tunnel: w455 -> [_ w479 _ w502 _ w536 _ w564 _]
                    tunnel: [FALSE FALSE FALSE FALSE FALSE FALSE FALSE FALSE TRUE] -> w454
                    tunnel: w453 -> [w461 _ w485 _ w512 _ w543 _ _]
                    tunnel: w452 -> [w460 _ w484 _ w511 _ w542 _ _]
                    frame "Turn Right 1" {
                      n302 = call "Auton Turn to disired angle.vi"("Power output range"=w461, "PID Turn  gains"=w460, "Angle setpoint"=35.0) -> ("In Range?"=w459:bool)  [unwired: 8 in]
                      n303 = Select(t=AutonEnumGoAround."Go Straight 1", s=w459, f=AutonEnumGoAround."Turn Right 1") -> (s? t:f=w464:T7)
                      n304 = case shown="True" w459 {
                        frame False {
                        }
                        frame True {
                          n305 = global read "Robot Values.vi" "Drive"() -> (w469:T10)
                          n306 = Bundle By Name(cluster=w469, "Drive Encoder reset"=TRUE) -> (w470:T10)
                          n307 = global write "Robot Values.vi" "Drive"(w470) -> ()
                          n308 = Wait (ms)(milliseconds to wait=u32 20) -> ()  [unwired: 1 out]
                        }
                      }
                    }
                    frame "Go Straight 1" {
                      n309 = call "Auton go linear distance.vi"("Average gains"=w479, "PID setpoint"=50.0, "Goal"=50.0, "output range"=w480) -> ("Done?"=w474:bool)  [unwired: 4 in]
                      n310 = Select(t=AutonEnumGoAround."Turn Left 1", s=w474, f=AutonEnumGoAround."Go Straight 1") -> (s? t:f=w478:T7)
                      n311 = global read "Robot Values.vi" "Drive"() -> (w472:T10)
                      n312 = Bundle By Name(cluster=w472, "Drive Encoder reset"=FALSE) -> (w473:T10)
                      n313 = global write "Robot Values.vi" "Drive"(w473) -> ()
                    }
                    frame "Turn Left 1" {
                      n314 = call "Auton Turn to disired angle.vi"("Power output range"=w485, "PID Turn  gains"=w484, "Angle setpoint"=-40.0) -> ("In Range?"=w483:bool)  [unwired: 8 in]
                      n315 = Select(t=AutonEnumGoAround."Go Straight 2", s=w483, f=AutonEnumGoAround."Turn Left 1") -> (s? t:f=w489:T7)
                      n316 = case shown="True" w483 {
                        frame False {
                        }
                        frame True {
                          n317 = global read "Robot Values.vi" "Drive"() -> (w493:T10)
                          n318 = Bundle By Name(cluster=w493, "Drive Encoder reset"=TRUE) -> (w494:T10)
                          n319 = global write "Robot Values.vi" "Drive"(w494) -> ()
                          n320 = Wait (ms)(milliseconds to wait=u32 20) -> ()  [unwired: 1 out]
                        }
                      }
                    }
                    frame "Go Straight 2" {
                      n321 = call "Auton go linear distance.vi"("Average gains"=w502, "PID setpoint"=81.0, "Goal"=78.0, "output range"=w501) -> ("Done?"=w498:bool)  [unwired: 4 in]
                      n322 = Select(t=AutonEnumGoAround."Turn Left 2", s=w498, f=AutonEnumGoAround."Go Straight 2") -> (s? t:f=w500:T7)
                      n323 = global read "Robot Values.vi" "Drive"() -> (w497:T10)
                      n324 = Bundle By Name(cluster=w497, "Drive Encoder reset"=FALSE) -> (w496:T10)
                      n325 = global write "Robot Values.vi" "Drive"(w496) -> ()
                    }
                    frame "Turn Left 2" {
                      # "Now a turn right"
                      n326 = global read "Robot Values.vi" "Lift System"() -> (w508:T11)
                      n327 = Bundle By Name(cluster=w508, "Lift Position"=2) -> (w509:T11)
                      n328 = global write "Robot Values.vi" "Lift System"(w509) -> ()
                      n329 = call "Auton Turn to disired angle.vi"("Power output range"=w512, "PID Turn  gains"=w511, "Angle setpoint"=-6.0) -> ("In Range?"=w510:bool)  [unwired: 8 in]
                      n330 = Select(t=AutonEnumGoAround."Go Straight 3", s=w510, f=AutonEnumGoAround."Turn Left 2") -> (s? t:f=w514:T7)
                      n331 = case shown="True" w510 {
                        frame False {
                        }
                        frame True {
                          n332 = global read "Robot Values.vi" "Drive"() -> (w521:T10)
                          n333 = Bundle By Name(cluster=w521, "Drive Encoder reset"=TRUE) -> (w520:T10)
                          n334 = global write "Robot Values.vi" "Drive"(w520) -> ()
                          n335 = Wait (ms)(milliseconds to wait=u32 20) -> ()  [unwired: 1 out]
                        }
                      }
                    }
                    frame "Go Straight 3" {
                      n336 = call "Auton go linear distance.vi"("Average gains"=w536, "PID setpoint"=77.0, "Goal"=77.0, "output range"=cluster{"output high":dbl, "output low":dbl} {"output high"=0.5, "output low"=-0.5}) -> ("Done?"=w533:bool)  [unwired: 4 in]
                      n337 = Select(t=AutonEnumGoAround."Nothing", s=w533, f=AutonEnumGoAround."Go Straight 3") -> (s? t:f=w535:T7)
                      n338 = global read "Robot Values.vi" "Lift System"() -> (w528:T11)
                      n339 = Bundle By Name(cluster=w528, "Lift Position"=2) -> (w529:T11)
                      n340 = global read "Robot Values.vi" "Tote Stopper Motors"() -> (w526:cluster{"RelayValue":T5, "RelayValue 2":T5})
                      n341 = Bundle By Name(cluster=w526, "RelayValue"=WPI_RelayValue."Reverse", "RelayValue 2"=WPI_RelayValue."Forward") -> (w523:cluster{"RelayValue":T5, "RelayValue 2":T5})
                      n342 = global write "Robot Values.vi" "Lift System"(w529) -> ()
                      n343 = global read "Robot Values.vi" "Drive"() -> (w531:T10)
                      n344 = Bundle By Name(cluster=w531, "Drive Encoder reset"=FALSE) -> (w532:T10)
                      n345 = global write "Robot Values.vi" "Tote Stopper Motors"(w523) -> ()
                      n346 = global write "Robot Values.vi" "Drive"(w532) -> ()
                    }
                    frame "Turn Right 3" {
                      # "Not in use"
                      n347 = call "Auton Turn to disired angle.vi"("Power output range"=w543, "PID Turn  gains"=w542, "Angle setpoint"=0.0) -> ("In Range?"=w541:bool)  [unwired: 8 in]
                      n348 = Select(t=AutonEnumGoAround."Go Straight 4", s=w541, f=AutonEnumGoAround."Turn Right 3") -> (s? t:f=w546:T7)
                      n349 = case shown="True" w541 {
                        frame False {
                        }
                        frame True {
                          n350 = global read "Robot Values.vi" "Drive"() -> (w551:T10)
                          n351 = Bundle By Name(cluster=w551, "Drive Encoder reset"=TRUE) -> (w552:T10)
                          n352 = global write "Robot Values.vi" "Drive"(w552) -> ()
                          n353 = Wait (ms)(milliseconds to wait=u32 20) -> ()  [unwired: 1 out]
                        }
                      }
                    }
                    frame "Go Straight 4" {
                      # "Not in use"
                      n354 = call "Auton go linear distance.vi"("Average gains"=w564, "PID setpoint"=30.0, "Goal"=30.0, "output range"=w563) -> ("Done?"=w557:bool)  [unwired: 4 in]
                      n355 = Select(t=AutonEnumGoAround."Nothing", s=w557, f=AutonEnumGoAround."Go Straight 4") -> (s? t:f=w562:T7)
                      n356 = global read "Robot Values.vi" "Lift System"() -> (w554:T11)
                      n357 = Bundle By Name(cluster=w554, "Lift Position"=2) -> (w553:T11)
                      n358 = global write "Robot Values.vi" "Lift System"(w553) -> ()
                      n359 = global read "Robot Values.vi" "Drive"() -> (w558:T10)
                      n360 = Bundle By Name(cluster=w558, "Drive Encoder reset"=FALSE) -> (w559:T10)
                      n361 = global write "Robot Values.vi" "Drive"(w559) -> ()
                    }
                    frame "Nothing", Default {
                    }
                  }
                }
                n362 = Select(t=AutonEnum."Stack", s=w448, f=AutonEnum."Go Around") -> (s? t:f=w445:T6)
              }
              frame "Stack" {
                # "Drop totes on top of new tote then pickup the new tote"
                n363 = flat-sequence {
                  tunnel: [w580] -> w570
                  frame #0 {
                    n364 = Wait (ms)(milliseconds to wait=u32 250) -> ()  [unwired: 1 out]
                  }
                  frame #1 {
                    # "Note: Time value might \nneed to be adjusted"
                    n365 = global read "Robot Values.vi" "Tote Stopper Motors"() -> (w574:cluster{"RelayValue":T5, "RelayValue 2":T5})
                    n366 = Bundle By Name(cluster=w574, "RelayValue"=WPI_RelayValue."Off", "RelayValue 2"=WPI_RelayValue."Off") -> (w575:cluster{"RelayValue":T5, "RelayValue 2":T5})
                    n367 = global read "Robot Values.vi" "Lift System"() -> (w578:T11)
                    n368 = Bundle By Name(cluster=w578, "Lift Position"=0) -> (w577:T11)
                    n369 = global write "Robot Values.vi" "Tote Stopper Motors"(w575) -> ()
                    n370 = Wait (ms)(milliseconds to wait=u32 1000) -> ()  [unwired: 1 out]
                    n371 = global write "Robot Values.vi" "Lift System"(w577) -> ()
                  }
                  frame #2 {
                    n372 = global read "Robot Values.vi" "Drive"() -> (w586:T10)
                    n373 = Bundle By Name(cluster=w586, "Drive Encoder reset"=FALSE) -> (w587:T10)
                    n374 = local read "Totes grabed"() -> (w584:i32)
                    n375 = local read "Total totes 4"() -> (w592:i32)
                    n376 = global read "Robot Values.vi" "Sensors"() -> (w589:T12)
                    n377 = global write "Robot Values.vi" "Drive"(w587) -> ()
                    n378 = Bundle By Name(cluster=w589, "Gyro Reset"=TRUE) -> (w590:T12)
                    n379 = Increment(x=w584) -> (x+1=w583:i32)
                    n380 = global write "Robot Values.vi" "Sensors"(w590) -> ()
                    n381 = local write "Totes grabed"(w583) -> ()
                    n382 = Equal?(x=w584, y=w592) -> (x = y?=w591:bool)
                    n383 = Select(t=AutonEnum."Turn", s=w591, f=AutonEnum."Go Around") -> (s? t:f=w580:T6)
                  }
                }
              }
              frame "To Auto" {
                n384 = call "Auton go linear distance.vi"("Average gains"=w600, "PID setpoint"=300.0, "Goal"=300.0 ("Max"), "output range"=w599) -> ("Done?"=w595:bool)  [unwired: 4 in]
                n385 = case shown="True" w595 {
                  frame False {
                  }
                  frame True {
                    n386 = global read "Robot Values.vi" "Drive"() -> (w602:T10)
                    n387 = Bundle By Name(cluster=w602, "Drive Encoder reset"=TRUE) -> (w604:T10)
                    n388 = global write "Robot Values.vi" "Drive"(w604) -> ()
                    n389 = Wait (ms)(milliseconds to wait=u32 20) -> ()  [unwired: 1 out]
                  }
                }
                n390 = Select(t=AutonEnum."Release Totes", s=w595, f=AutonEnum."To Auto") -> (s? t:f=w596:T6)
              }
              frame "Release Totes" {
                w605 = -0.4
                n391 = global read "Robot Values.vi" "Tote Stopper Motors"() -> (w612:cluster{"RelayValue":T5, "RelayValue 2":T5})
                n392 = Bundle By Name(cluster=w612, "RelayValue"=WPI_RelayValue."Forward", "RelayValue 2"=WPI_RelayValue."Reverse") -> (w609:cluster{"RelayValue":T5, "RelayValue 2":T5})
                n393 = global write "Robot Values.vi" "Tote Stopper Motors"(w609) -> ()
                n394 = global read "DriveGlobal.vi" "Drive speeds"() -> (w606:T9)
                n395 = Bundle By Name(cluster=w606, "RightMotorSpeed"=w605, "LeftMotorSpeed"=w605) -> (w607:T9)
                n396 = global write "DriveGlobal.vi" "Drive speeds"(w607) -> ()
                n397 = Wait (ms)(milliseconds to wait=u32 1000) -> ()  [unwired: 1 out]
              }
              frame "Start" {
                w630 = TRUE  # Is finished
                # "Selector is left in case testing fails\nand it needs to switch."
                # "Will switch to push state after starting to\nlift the tote."
                # "Is finished is set to true because\nthe robot will lift the tote while\nit is moving forawrd in the\n\"Push\" state.\n\nThis still needs to be tested.\nAnother possible solution is a\ntimed delay if simoultaneous\ntesting fails."
                # "Grab and then lift first tote"
                n398 = global read "Robot Values.vi" "Tote Stopper Motors"() -> (w617:cluster{"RelayValue":T5, "RelayValue 2":T5})
                n399 = Bundle By Name(cluster=w617, "RelayValue"=WPI_RelayValue."Off", "RelayValue 2"=WPI_RelayValue."Off") -> (w614:cluster{"RelayValue":T5, "RelayValue 2":T5})
                n400 = global write "Robot Values.vi" "Tote Stopper Motors"(w614) -> ()
                n401 = global read "Robot Values.vi" "Sensors"() -> (w622:T12)
                n402 = Bundle By Name(cluster=w622, "Gyro Reset"=FALSE) -> (w623:T12)
                n403 = global write "Robot Values.vi" "Sensors"(w623) -> ()
                n404 = Wait (ms)(milliseconds to wait=u32 50) -> ()  [unwired: 1 out]
                n405 = global read "Robot Values.vi" "Drive"() -> (w628:T10)
                n406 = Bundle By Name(cluster=w628, "Drive Encoder reset"=FALSE) -> (w629:T10)
                n407 = global write "Robot Values.vi" "Drive"(w629) -> ()
                n408 = Select(t=AutonEnum."Go Around", s=w630, f=AutonEnum."Start") -> (s? t:f=w631:T6)
                n409 = global read "Robot Values.vi" "Lift System"() -> (w619:T11)
                n410 = Bundle By Name(cluster=w619, "Lift Position"=0) -> (w618:T11)
                n411 = case shown="True" w630 {
                  frame False {
                  }
                  frame True {
                    n412 = local read "Totes grabed"() -> (w633:i32)
                    n413 = Increment(x=w633) -> (x+1=w632:i32)
                    n414 = local write "Totes grabed"(w632) -> ()
                  }
                }
                n415 = global write "Robot Values.vi" "Lift System"(w618) -> ()
              }
              frame "Nothing", Default {
                # "Do nothing, this should never be reached unless an error has occured.\nIf an error has occured, this case should activate and stop the robot\nto prevent failure."
              }
            }
          }
          "Total totes 4" <- 1 ("Total totes")
        }
      }
      "Totes grabed" <- 0 ("Totes grabed")
    }
    frame Disabled {
      n416 = while {
        shift-right: [w637] -> _
        shift-left: Auton1ToteEnum."First Forward" -> [w638]
        stop <- FALSE stop-if-true
        n417 = case shown="\"First Forward\"" w638 {
          selector: w638 -> [_ _ _ w661 w666]
          tunnel: [Auton1ToteEnum."First Forward" w651 Auton1ToteEnum."First Pick Up" w661 w666] -> w637
          frame "Start", Default {
            n418 = global read "Robot Values.vi" "Lift System"() -> (w643:T11)
            n419 = Bundle By Name(cluster=w643, "Lift Position"=2) -> (w642:T11)
            n420 = global write "Robot Values.vi" "Lift System"(w642) -> ()
            n421 = Wait (ms)(milliseconds to wait=u32 5000) -> ()  [unwired: 1 out]
          }
          frame "First Forward" {
            n422 = call "Auton go linear distance.vi"("Average gains"="Average gains", "PID setpoint"=254.0 ("setpoint"), "Goal"=254.0 ("y"), "output range"=cluster{"output high":dbl, "output low":dbl} {"output high"=0.35, "output low"=-0.35}) -> ("Done?"=w644:bool)  [unwired: 4 in]
            n423 = Select(t=Auton1ToteEnum."Get First Tote", s=w644, f=Auton1ToteEnum."First Forward") -> (s? t:f=w651:T8)
          }
          frame "Get First Tote" {
            n424 = global read "Robot Values.vi" "Lift System"() -> (w660:T11)
            n425 = Bundle By Name(cluster=w660, "Lift Position"=0) -> (w659:T11)
            n426 = global write "Robot Values.vi" "Lift System"(w659) -> ()
            n427 = global read "DriveGlobal.vi" "Drive speeds"() -> (w657:T9)
            n428 = Bundle By Name(cluster=w657, "RightMotorSpeed"=0.0, "LeftMotorSpeed"=0.0) -> (w656:T9)
            n429 = global write "DriveGlobal.vi" "Drive speeds"(w656) -> ()
            n430 = Wait (ms)(milliseconds to wait=u32 50) -> ()  [unwired: 1 out]
          }
          frame "First Pick Up" {
            n431 = global read "Robot Values.vi" "Lift System"() -> (w664:T11)
            n432 = Bundle By Name(cluster=w664, "Lift Position"=1) -> (w663:T11)
            n433 = global write "Robot Values.vi" "Lift System"(w663) -> ()
            n434 = Wait (ms)(milliseconds to wait=u32 50) -> ()  [unwired: 1 out]
          }
          frame "Stop" {
          }
        }
      }
    }
  }
  n435 = while {
    stop <- FALSE stop-if-true
    n436 = call <vilib>:"WPI_DriverStationReport Robot Code State.vi"("Autonomous"=TRUE) -> ()  [unwired: 10 in, 1 out]
    n437 = Wait (ms)(milliseconds to wait=u32 20) -> ()  [unwired: 1 out]
  }
  n438 = call <vilib>:"WPI_DriverStationGet Alliance Info.vi"() -> ()  [unwired: 12 out]
  n439 = call <vilib>:"WPI_JoystickRefNum Registry Get.vi"("refnum name"="Joystick 0") -> ("JoystickDevRef"=w3:T13)  [unwired: 1 in, 9 out]
  n440 = call <vilib>:"WPI_JoystickGetValues.vi"("JoystickDevRef"=w3) -> ("Axes"=w1:dbl[])  [unwired: 6 in, 4 out]
  n441 = call <vilib>:"SD Write Numeric Array.vi"("Numeric Array"=w1, "Name"="Joystick 0/Axes") -> ()  [unwired: 8 in, 2 out]
  n442 = disable-structure shown="Disabled" {
    frame Disabled {
      w673 = "RobotDrive Motors" ("Name")
      # "This is some simple sample code to drive your robot curving one direction and then the other."
      # "stand still"
      # "turn left for 0.5 second"
      # "turn right for 1 second"
      n443 = call <vilib>:"WPI_RobotDriveRefNum Registry Get.vi"("refnum name"="Left and Right Motors") -> ("RobotDriveDevRef"=w674:T15)  [unwired: 1 in, 9 out]
      n444 = call-poly <vilib>:"WPI_RobotDriveArcadeDrive.vi"("Y axis value"=0.5 ("X axis value"), "X axis value"=0.25, "RobotDriveDevRef"=w674) -> ("Motor Values"=w672:dbl[], "RobotDriveDevRef"=w681:T15)  [unwired: 1 in, 6 out]
      n445 = call-poly <vilib>:"SD Write Value.vi"("Numeric Array"=w672, "Name"=w673) -> ()  [unwired: 8 in, 2 out]
      n446 = call <vilib>:"WPI_RobotDriveDelayAndUpdateSafety.vi"("Delay (s)"=1.0, "RobotDriveDevRef"=w681) -> ("RobotDriveDevRef 2"=w680:T15)  [unwired: 8 in, 1 out]
      n447 = call-poly <vilib>:"WPI_RobotDriveArcadeDrive.vi"("Y axis value"=0.25 ("X axis value"), "X axis value"=0.5, "RobotDriveDevRef"=w680) -> ("Motor Values"=w671:dbl[], "RobotDriveDevRef"=w679:T15)  [unwired: 1 in, 6 out]
      n448 = call-poly <vilib>:"SD Write Value.vi"("Numeric Array"=w671, "Name"=w673) -> ()  [unwired: 8 in, 2 out]
      n449 = call <vilib>:"WPI_RobotDriveDelayAndUpdateSafety.vi"("Delay (s)"=0.5, "RobotDriveDevRef"=w679) -> ("RobotDriveDevRef 2"=w678:T15)  [unwired: 8 in, 1 out]
      n450 = call-poly <vilib>:"WPI_RobotDriveArcadeDrive.vi"("Y axis value"=0.0 ("X axis value"), "X axis value"=0.0, "RobotDriveDevRef"=w678) -> ("Motor Values"=w670:dbl[])  [unwired: 1 in, 7 out]
      n451 = call-poly <vilib>:"SD Write Value.vi"("Numeric Array"=w670, "Name"=w673) -> ()  [unwired: 8 in, 2 out]
    }
    frame Enabled {
    }
  }
  n452 = disable-structure shown="Disabled" {
    frame Disabled {
      # "This sample code describes robot movements in an array. You can extend it to control other motors\non your robot. You can also use file I/O to move the data to a text file."
      n453 = call <vilib>:"WPI_RobotDriveRefNum Registry Get.vi"("refnum name"="Left and Right Motors") -> ("RobotDriveDevRef"=w689:T15)  [unwired: 1 in, 9 out]
      n454 = for {
        shift-right: [w696] -> _
        shift-left: w689 -> [w697]
        tunnel: "Array of robot movements" -> [w692] mode=indexing
        n455 = Unbundle By Name(w692) -> ("X Joystick Value"=w695:dbl, "Y Joystick Value"=w694:dbl, "Delay (sec)"=w693:dbl)  [unwired: 1 out]
        n456 = call-poly <vilib>:"WPI_RobotDriveArcadeDrive.vi"("Y axis value"=w694, "X axis value"=w695, "RobotDriveDevRef"=w697) -> ("Motor Values"=w691:dbl[], "RobotDriveDevRef"=w698:T15)  [unwired: 1 in, 6 out]
        n457 = call-poly <vilib>:"SD Write Value.vi"("Numeric Array"=w691, "Name"="RobotDrive Motors") -> ()  [unwired: 8 in, 2 out]
        n458 = call <vilib>:"WPI_RobotDriveDelayAndUpdateSafety.vi"("Delay (s)"=w693, "RobotDriveDevRef"=w698) -> ("RobotDriveDevRef 2"=w696:T15)  [unwired: 8 in, 1 out]
        "Current Movement, for debugging" <- w692
      }
    }
    frame Enabled {
    }
  }
  n459 = Default Directory() -> ()  [unwired: 1 out]
